vi "AlliGator GUI Actions.vi"(0 "AlliGator Q Elements in":T4[](array[typedef]), 1 "VI in":refnum<vi>, 2 "Script":bool, 5 "AlliGator IV DVR":refnum<data-value>, 7 "AlliGator Q Event in":T5=enum."GUI:Idle", 9 "Data":variant, 11 "error in (no error)":errorcluster, 12 "AlliGator Ctrl Refnums":T6) -> (3 "Script?":bool, 4 "AlliGator Q Elements out":T4[](array[typedef]), 6 "AlliGator IV DVR":refnum<data-value>, 10 "[Notebook Message]":T1[](array[typedef]) {"Message Style"."Text Alignment" items=["Left", "Right", "Center"]}, 14 "Quit?":bool, 15 "error out":errorcluster)   [LabVIEW 2021, in "AlliGator Action Engine.lvlib"]
doc: "Processes AlliGator GUI-related actions."
uses:
  AlliGator Action Engine.lvlib
  AlliGator Displayed Image.ctl
  AlliGator Source Image.lvlib
  Alligator Elements Order in Action Stack.ctl
  AlliGator Q Event.ctl
  AlliGator Q Element.ctl
  AlliGator GUI.lvlib
  AlliGator Variables List.ctl
  AlliGator Globals, Variables & Constants.lvlib
  Variant/Variant to Data/Variant to Data.lvlib
  Variant/Variant to Data/Variant to U16.vi
  AlliGator Internal Variables.lvlib
  GUI/Embedded Progress Bar Q Element.ctl
  GUI/GUI.lvlib
  AlliGator ROIs.lvlib
  Rich Text Box/Rich Text Box.lvlib
  Strings/Strings.lvlib
  AlliGator Settings.lvlib
  Notebook/Notebook.lvlib
  AlliGator Scripts.lvlib
  Variant/Variant to Data/Variant to Boolean.vi
  AlliGator Settings List.ctl
  AlliGator Abort.vi
  AlliGator State Indicators List.ctl
  AlliGator Set State Indicator Data.ctl
  AlliGator Globals.vi
  Variant/Variant to Data/Variant to String.vi
  AlliGator Python Plugins.lvlib
  Fits/Abort Fit Global.vi
  Fits/Fits.lvlib
  Utilities/Utilities.lvlib
  GUI/Open VI Options.ctl
  AlliGator Windows List.ctl
  AlliGator Open Wndow Event Data.ctl
  Sound/Sound.lvlib
  Formula/Formula.lvlib
  Variant/Variant to Data/Variant to I32.vi
  Test Suites/AlliGator Test Data.ctl
  Test Suites/AlliGator Test Suite.lvlib
  Phasor/Phasor Reference Series.ctl
  Phasor/Phasor.lvlib
  Phasor/Calibration Phasor (m, phi).ctl
  Phasor/Phasor (g, s).ctl
  <vilib>/vision/Image Controls.llb/IMAQ Image.ctl
  Image/Named ROI Description.ctl
  Image/Image.lvlib
  AlliGator Baseline Subtraction Method.ctl
  AlliGator Decay Preprocessing.lvlib
  AlliGator Decay Background Subtraction Info.ctl
  Graphs/XY Graph/XY Graph Plot Shift Method.ctl
  Graphs/XY Graph/XY Graph Add-Ons.lvlib
  Graphs/XY Graph/XY Graph Plot Shift Parameters.ctl
  AlliGator Decay Extrapolation Parameters.ctl
  AlliGator Decay Metadata v3.ctl
  AlliGator Phasor Graph.lvlib
  AlliGator Raw Phasor Plot Data v4.ctl
  AlliGator Data Series Type.ctl
  AlliGator Files.lvlib
  AlliGator Gate Image Set.ctl
  AlliGator FLI Dataset Type.ctl
  Phasor/Phasor Harmonic Data.ctl
  AlliGator Phasor Multi-Harmonic Data.ctl
  AlliGator Phasor Plot.lvlib
  Fits/IRF(X)PSED/Decay Fit Parameters & Derived Quantities List.ctl
  Fits/IRF(X)PSED/Decay Fit Parameters In List.ctl
  AlliGator Decay Fit Parameter Constraints 2.ctl
  AlliGator Decay Fit.lvlib
  Fits/Decay Convolution/Decay Model.ctl
  Fits/Residual Type.ctl
  Fits/IRF(X)PSED/Fit Weights Type.ctl
  Fits/Fit Calculation Method.ctl
  Fits/Non-linear Fitting Algorithm.ctl
  AlliGator Decay Fit Options & Parameters v2.ctl
  AlliGator Decay Fit Parameter Map.lvlib
  AlliGator Gate Arithmetic.ctl
  AlliGator Internal Variables v2.ctl
  AlliGator Registered Events Ctrl Refnums.ctl
  AlliGator Dataset Ctrl Refnums.ctl
  Phasor/Phasor Calibration Type.ctl
  AlliGator Phasor Graph Ctrl Refnums.ctl
  AlliGator Phasor Plot Ctrl Refnums.ctl
  AlliGator State Indicator.ctl
  AlliGator Other Ctrl Refnums.ctl
  AlliGator Image Histogram Control Refnums.ctl
  AlliGator Decay Fit Map Control Refnums.ctl
  AlliGator Ctrl Refnums.ctl
  Rich Text Box/Text Colors.ctl
  Rich Text Box/Text Formatting.ctl
  AlliGator Dataset Channel.ctl
  AlliGator Dual-Channel Datasets.lvlib
  Histograms/Histogram Bin Position.ctl
  Histograms/Histogram Window.lvlib
  Histograms/Histogram Bin Option.ctl
  Histograms/Linear Histogram Options.ctl
  AlliGator Decay Preprocessing Parameters.ctl
  Phasor/Phasor Standard Deviation Options.ctl
  Phasor/Phasor Calibration Map v2.ctl
  Fits/Non-linear Fitting Method v2.ctl
  Fits/IRF(X)PSED/Decay Fit Options v2.ctl
  Fits/IRF(X)PSED/MLE Baseline Offset Type.ctl
  Notebook/Notebook Message Object.ctl
  AlliGator Parameter Maps Data.ctl
  AlliGator Main Window Tabs.ctl
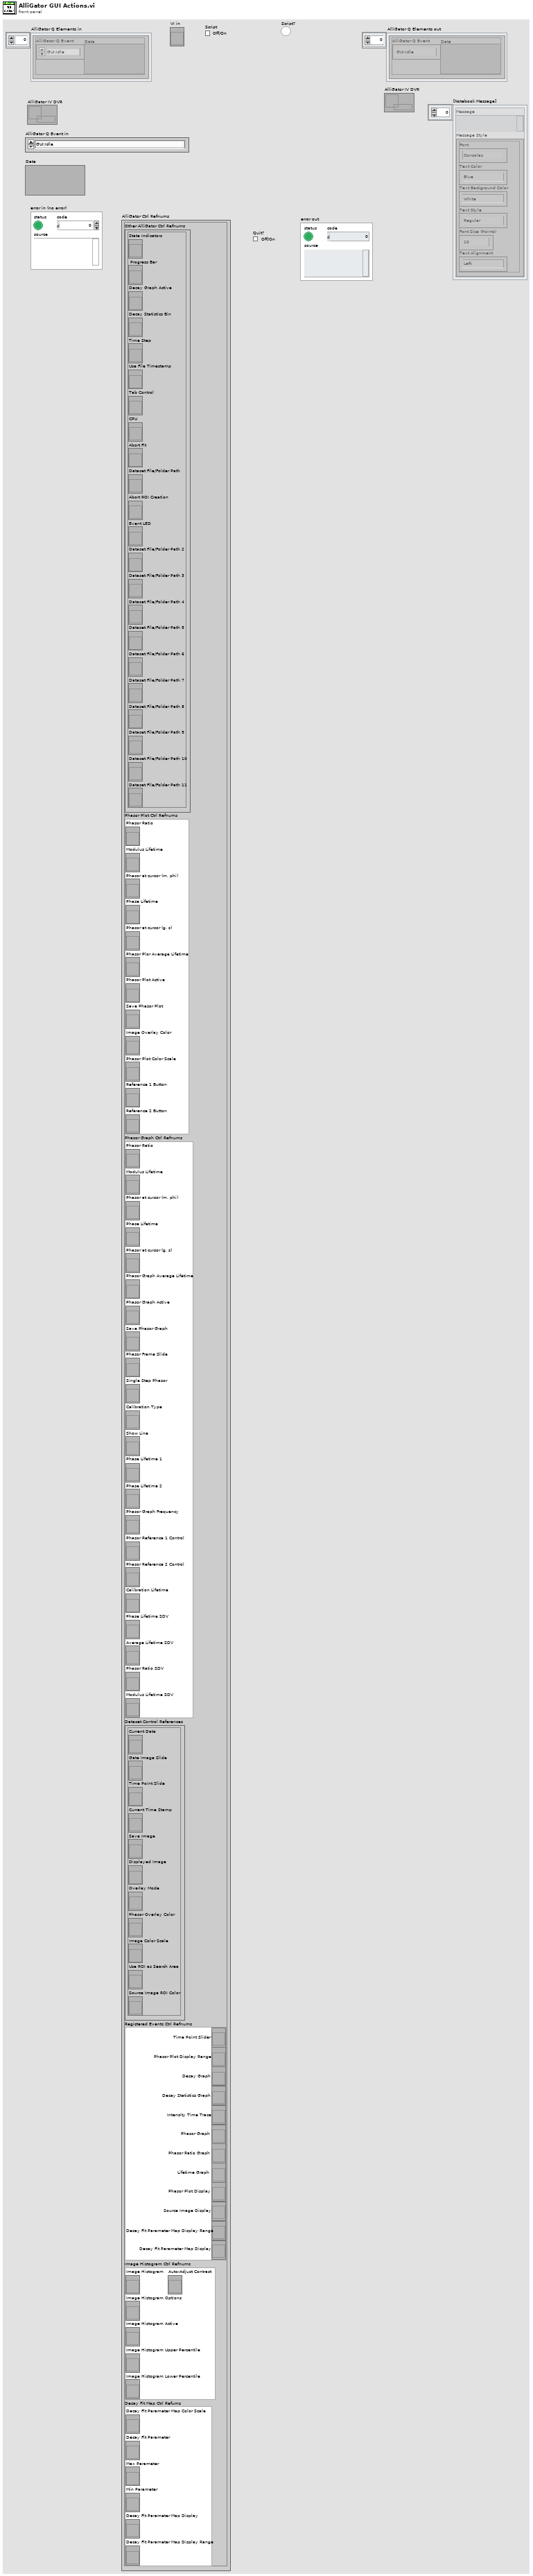
[diagram p1: front panel]
types:
  T1 = typedef "Notebook.lvlib/Notebook Message Object.ctl" = cluster{"Message":string, "Message Style":T2}
  T2 = typedef "Rich Text Box.lvlib/Text Formatting.ctl" = cluster{"Font":string, "Text Color":T3, "Text Background Color":T3, "Text Style":enum16{"Regular", "Bold", "Italic", "Underline", "Strikeout"}, "Font Size (Points)":dbl, "Text Alignment":i32}
  T3 = typedef "Rich Text Box.lvlib/Text Colors.ctl" = enum16{"Unchanged", "Black", "Blue", "Brown", "Gray", "Green", "Orange", "Pink", "Red", "White"}
  T4 = typedef "AlliGator Action Engine.lvlib/AlliGator Q Element.ctl" = cluster{"AlliGator Q Event":T5, "Data":variant}
  T5 = typedef "AlliGator Action Engine.lvlib/AlliGator Q Event.ctl" = enum16{"---- Files ----", "Files:Set Batch Export Files To Save", "Files:Set Dataset Loading & Pre-processing Options", "Files:Check #Frames in Dataset", "Files:Increment Frame Index", "Files:Open Mask Image", "Files:Open White Light Image", "Files:Open Single Dataset", "Files:New Folder of Folders Selected", "Files:Load File (all Types)_Scriptable", "Files:Move Flattened Series to Folders Series", "Files:Select Folder", "Files:Load FLI Dataset", "Files:Load Swiss SPAD 1 Dataset", "Files:Load Swiss SPAD 2 Dataset", "Files:Load .sdt FLI Dataset", "Files:Load .ptu FLI Dataset", "Files:Load .bin FLI Dataset", "Files:Load Single Gate Image Folder", "Files:Load I/m/phi Dataset (deprecated)", "Files:Load Single Image", "Files:Subtract Background File", "Files:Export FLI Dataset", "Files:Load HDF5 FLI Dataset", "Files:Set Destination File Path", "Files:Save Mask Image", "Files:Batch Conversion", "Files:New Folder Selected", "Files:Close FLI Dataset", "Files:Close FLI Dataset Series", "Files:Close White Light Image", "Files:Close Mask Image", "---- FLI Dataset ----", "FLI Dataset:Channel Arithmetic", "FLI Dataset:Export Average Lifetime Map as ASCII", "FLI Dataset:Export User-Defined Quantity Map as ASCII", "FLI Dataset:Python Function FLI Dataset Event", "FLI Dataset:ROI Analysis", "FLI Dataset:Tilted Logistic Square Gated IRF Characteristics Map", "FLI Dataset:Logistic Square Gated IRF Characteristics Map", "FLI Dataset:Square Gated IRF Characteristics Map", "FLI Dataset:Multi-ROI Single-Pixel Phasor Analysis", "FLI Dataset:Multi-ROI Single-Pixel NLSF Analysis", "FLI Dataset:All ROIs IRF Extraction", "FLI Dataset:All ROIs Decay Fit Non-Interactive (Fast + Individual IRF)", "FLI Dataset:All ROIs Phasor Analysis", "FLI Dataset:All ROIs Decay Fit", "FLI Dataset:Fluorescence Decay Statistics", "FLI Dataset:Update Decay Statistics Graph", "FLI Dataset:Get Decay from ROI", "FLI Dataset:All ROIs Average Lifetimes", "---- FLI Dataset Series ----", "FLI Dataset Series:Sum All Datasets in Series", "FLI Dataset Series:Add Dataset to Accumulated Dataset", "FLI Dataset Series:Display Accumulated Dataset", "FLI Dataset Series:Clear Dataset Series Sum", "FLI Dataset Series:Time-Series Analysis (NLSF)", "FLI Dataset Series:Time-Series Analysis (Phasor)", "---- Image ----", "Image:Update Image Profile Plots", "Image:Image Histogram Cursor Move", "Image:Image Histogram", "Image:Image Contrast", "Image:Set Image Histogram Cursor Move Flag", "Image:Clear Image Overlay", "Image:Use ROI as Search Area", "Image:Set ROI Diameter", "Image:Save Image Data as TIFF", "Image:Save Displayed Image with Overlay", "Image:Save Image Overlay Only", "Image:Save Image as Hot Pixel Mask", "Image:Change Source Image Color Palette", "Image:Copy Image to Clipboard", "Image:Source Image ROI Selection", "Image:Delete All ROIs", "Image:Delete All Unselected ROIs", "Image:Delete ROI", "Image:Merge All ROIs", "Image:Store ROI", "Image:Source Image ROI Storage", "Image:Export ROI Description to Notebook", "Image:Save ROI", "Image:Load ROI", "Image:Paste ROI Definition", "Image:Clear ROI", "Image:Identify ROIs in Mask Image", "Image:Create Complementary ROI", "Image:Create Contour ROI", "Image:Create ROI(s) from Pixels with Peak above Min_Scriptable", "Image:Create ROI(s) from Pixels with Intensity above Min_Scriptable", "Image:Compute ROI Statistics", "Image:Delete ROI(s) based on ROI Characteristics", "Image:Create ROI Grid", "Image:ROI to Individual Pixel ROIs", "Image:Python Function Source Image Event", "Image:Show Phasor Calibration Map ROI Centers", "Image:Convert ROI to Mask Image", "Image:Mouse Move", "Image:Mouse Up", "Image:Set Source Image Mouse Move Flag", "Image:Add Scale Bar Overlay", "Image:Delete Existing ROIs Option", "---- Decay ----", "Decay:Clear IRF/Reference Plot", "Decay:Clear Local IRFs", "Decay:Add Decay to Graph", "Decay:Smoothen Plot", "Decay:Smoothen Plot Tail", "Decay:Average Selected Plots", "Decay:Extract IRF", "Decay:Optimal IRF Extraction", "Decay:Threshold IRF", "Decay:Fit to Model IRF", "Decay:Fit IRF to Square Gate", "Decay:Fit IRF to Logistic Square Gate", "Decay:Fit IRF to Tilted Logistic Square Gate", "Decay:Create Bounding Cursors Set", "Decay:Export Bounding Cursors Definition to Notebook", "Decay:Denoise Plot", "Decay:Compute Cumulative Function", "Decay:Use as Reference Decay", "Decay:Show Reference Decay/IRF", "Decay:Extrapolate Decay", "Decay:Create Head & Tail Bounding Cursors", "Decay:Store Cursor-defined Head & Tail Fractions", "Decay:Rebin Plot", "Decay:1-Normalize Decay", "Decay:[0-1]-Normalize Plot", "Decay:Straighten Decay", "Decay:Shift Decay", "Decay:Fold Decay", "Decay:Fit Decay", "Decay:Global Fit of Selected Decays", "Decay:Post Global Fit Script", "Decay:Add Global Fit Parameters to Graph", "Decay:Add Decay Parameter(s) to Plot (Graph)", "Decay:Export Decay to Phasor Graph", "Decay:Plot Decay Shifts", "Decay:Compute Average Lifetime", "Decay:Plot Convolution", "Decay:Graph Tip Strip Update", "---- Decay Statistics ----", "Decay Statistics:Tip Strip Update", "---- Intensity Time Trace ----", "Intensity Time Trace:Use File Timestamp", "Intensity Time Trace:Load Intensity Corrections File", "Intensity Time Trace:Clear Intensity Corrections File", "Intensity Time Trace:Tip Strip Update", "---- Phasor Plot ----", "Phasor Plot:Build Phasor Plot", "Phasor Plot:Change Phasor Plot Color Palette", "Phasor Plot:Adjust Phasor Plot Display Range", "Phasor Plot:Highlight Image ROI in Phasor Plot", "Phasor Plot:Save Phasor Plot Image with Overlay", "Phasor Plot:Export Complex Phasor Map", "Phasor Plot:Export Phasor Ratio Map", "Phasor Plot:Export Average Lifetime Map", "Phasor Plot:Compute Phase Lifetime Histogram", "Phasor Plot:Compute Phasor Ratio Histogram", "Phasor Plot:Compute Phase Lifetime vs Intensity Scatter Plot", "Phasor Plot:Weber 2-Component Decomposition", "Phasor Plot:Update Phasor Color Map Vertices", "Phasor Plot:Clear Phasor Overlay", "Phasor Plot:Use Segment Extremities as References", "Phasor Plot:Use UC/Segment Intersections as References", "Phasor Plot:Use UC/Principal Axis Intersections as References", "Phasor Plot:Use UC/Linear Fit Intersections as References", "Phasor Plot:Update Phasor Plot Reference", "Phasor Plot:Show Local Phasor Info in Phasor Plot", "Phasor Plot:Update Phasor Plot State", "Phasor Plot:Phasor Plot ROI Storage", "Phasor Plot:Phasor Plot ROI Selection", "Phasor Plot:Python Function Phasor Plot Event", "Phasor Plot:Overlay Phasor ROI, Ratio or Map in Source Image", "Phasor Plot:Compute Decay of Selected Phasors", "Phasor Plot:Phasor at Image Pixel", "Phasor Plot:Mouse Move", "Phasor Plot:Mouse Up", "Phasor Plot:Display Range Mouse Move", "Phasor Plot:Set Mouse Move Flag", "---- Phasor Graph ----", "Phasor Graph:Calibrated Phasor Map Series", "Phasor Graph:Whole Image Phasor Scatter Plot (Todo)", "Phasor Graph:Get Phasor Value", "Phasor Graph:Create New Phasor Plot Dialog", "Phasor Graph:Update Last Phasor Value", "Phasor Graph:Update Phasor (m, phi)", "Phasor Graph:Remove Single Phasor from Plot", "Phasor Graph:Add Single Phasor to Plot", "Phasor Graph:Remove Phasor Plot", "Phasor Graph:Remove Selected Phasor Plots", "Phasor Graph:Clear Phasor Data", "Phasor Graph:Clear Phasor Graph", "Phasor Graph:Cursor Move", "Phasor Graph:Draw Cursor Connecting Line", "Phasor Graph:Clear Cursor Connecting Line", "Phasor Graph:Find UC Intersection", "Phasor Graph:Use UC/Cursor-Defined Line Intersections", "Phasor Graph:Use Selected Plots Fitted Line/UC Intersections", "Phasor Graph:Use Selected Plots Principal Axis/UC Intersections", "Phasor Graph:Show Single Phasor", "Phasor Graph:Save Single Phasor Plot", "Phasor Graph:Save All Phasor Plots", "Phasor Graph:Load Phasor Plot(s)", "Phasor Graph:Phasor Multiplication", "Phasor Graph:Compute Average Phasor", "Phasor Graph:Compute Multiple Average Phasors (Selected Plots)", "Phasor Graph:Export Single Phasor Plot Phase Lifetimes", "Phasor Graph:Phase Lifetime Trajectory", "Phasor Graph:Phase Lifetime vs Intensity Scatter Plot (deprecated)", "Phasor Graph:Parameter 2 vs Parameter 1 Scatter Plot", "Phasor Graph:Use Cursor n Location", "Phasor Graph:Set Reference n to Current Phase Lifetime Value", "Phasor Graph:Set Reference n to Lifetime Value", "Phasor Graph:Set Cursor n Location", "Phasor Graph:Save Phasor Graph Image", "Phasor Graph:Update SEPL Plot", "Phasor Graph:Export Single Phasor Plot Data", "Phasor Graph:Export Selected Phasor Plots Data", "Phasor Graph:Python Function Phasor Graph Event", "Phasor Graph:Tip Strip Update", "---- Calibration ----", "Calibration:Set Calibration Type", "Calibration:Load/Save Phasor Calibration", "Calibration:Load/Save Phasor Calibration Series", "Calibration:Load/Save Phasor Calibration Map", "Calibration:Use as Calibration", "Calibration:Compute Optimal Calibration from Phasor References", "Calibration:Clear Phasor Calibration", "Calibration:Single Phasor Calibration Information", "Calibration:Use as Calibration Series", "Calibration:Use as Calibration Map", "Calibration:Clear Calibration Series", "Calibration:Phasor Calibration Series Information", "Calibration:Clear Calibration Map", "Calibration:Phasor Calibration Map Information", "Calibration:Apply Phasor Calibration", "Calibration:Update Single Plot Calibration", "Calibration:Update Multiple Plots Calibration", "Calibration:Clear Single Plot Calibration", "Calibration:Clear All Plots Calibrations", "Calibration:Clear Plot(s) Calibration(s)?", "Calibration:Phasor Calibration Maps (# Gates Series)", "---- Phasor Ratio ----", "Phasor Ratio:Clear Reference n", "Phasor Ratio:Toggle Selected Plot(s)  Lock to Reference 1", "Phasor Ratio:Use as Reference n", "Phasor Ratio:Send Reference n to Notebook", "Phasor Ratio:Toggle Selected Plot(s)  Lock to Reference 2", "Phasor Ratio:Compute Phasor Ratio at Mouse Location", "Phasor Ratio:Compute Phasor Plot's Average Phasor Ratio", "Phasor Ratio:Compute Time-Series Phasor Ratios", "Phasor Ratio:Fit Line to Phasor Ratio Plot", "Phasor Ratio:Save References", "Phasor Ratio:Load References", "Phasor Ratio:Update Phasor Reference 1", "Phasor Ratio:Update Phasor Reference 2", "Phasor Ratio:Move Cursor n to Reference n", "Phasor Ratio:Use as Phasor Reference 1 Lifetime", "Phasor Ratio:Use as Phasor Reference 2 Lifetime", "Phasor Ratio:Export Phasor Ratio Map as ASCII", "Phasor Ratio:Tip Strip Update", "---- Lifetime & Other Parameters Graph ----", "Lifetime:Tip Strip Update", "---- Decay Fit Parameter Map ----", "Decay Fit Parameter Map:Export ROI NLSF Data as ASCII", "Decay Fit Parameter Map:Set Decay Fit  Parameter Map Selection", "Decay Fit Parameter Map:Build Decay Fit Parameter Map", "Decay Fit Parameter Map:Change Decay Fit Parameter Map Color Palette", "Decay Fit Parameter Map:Export Decay Fit Parameter Map Data as ASCII", "Decay Fit Parameter Map:Export All Decay Fit Parameter Maps Data as ASCII", "Decay Fit Parameter Map:Send Map Data to Lifetime Graph", "Decay Fit Parameter Map:Save Decay Fit Parameter Map Image", "Decay Fit Parameter Map:Save-Load IRFs & Fit Data", "Decay Fit Parameter Map:Update Local Decay Plots", "Decay Fit Parameter Map:Python Function Decay Fit Parameters Map Event", "Decay Fit Parameter Map:Overlay Decay Fit Parameter Map in Source Image", "Decay Fit Parameter Map:Plot Map Data vs Intensity", "Decay Fit Parameter Map:Mouse Up", "Decay Fit Parameter Map:Display Range Mouse Move", "---- Generic Graph ----", "Generic Graph:Generic XY Graph Event", "Generic Graph:Python Function XY Graph Event", "Generic Graph:New Plot", "Generic Graph:Save Plot", "Generic Graph:XY Plot Histogram", "Generic Graph:Set XY Graph Plot Name", "Generic Graph:Set Last Cursor Style", "Generic Graph:Tip Strip Update", "---- GUI ----", "GUI:Start Script", "GUI:Type of Displayed Image Changed", "GUI:Gate Image Slide Changed", "GUI:Show Busy Icon", "GUI:Show Busy Icon & Abort Button", "GUI:Hide Busy Icon", "GUI:Hide Busy Icon & Abort Button", "GUI:Abort", "GUI:End Script", "GUI:Start Timing", "GUI:End Timing", "GUI:Set State Indicator", "GUI:Send Parameters JSON Strings to Clipboard", "GUI:Set Gate Step", "GUI:Idle", "GUI:Initialization", "GUI:Quit", "GUI:Increment Dataset Index", "GUI:Set Dataset Index to -1", "GUI:Time Series Slider Moved", "GUI:Time Series Slider Changed", "GUI:Toggle Playback or Loop", "GUI:Playback Script", "GUI:Set Phasor Frequency", "GUI:Open Window", "GUI:Start Test Script", "GUI:End Test Script", "DEBUG"}
  T6 = typedef "AlliGator GUI.lvlib/AlliGator Ctrl Refnums.ctl" = cluster{"Other AlliGator Ctrl Refnums":T7, "Phasor Plot Ctrl Refnums":T8, "Phasor Graph Ctrl Refnums":T9, "Dataset Control References":T10, "Registered Events Ctrl Refnums":T11, "Image Histogram Ctrl Refnums":T12, "Decay Fit Map Ctrl Refums":T13}
  T7 = typedef "AlliGator GUI.lvlib/AlliGator Other Ctrl Refnums.ctl" = cluster{"State Indicators":refnum<vi>, " Progress Bar":refnum<vi>, "Decay Graph Active":refnum<vi>, "Decay Statistics Bin":refnum<vi>, "Time Step":refnum<vi>, "Use File Timestamp":refnum<vi>, "Tab Control":refnum<vi>, "CPU":refnum<vi>, "Abort Fit":refnum<vi>, "Dataset File/Folder Path":refnum<vi>, "Abort ROI Creation":refnum<vi>, "Event LED":refnum<vi>, "Dataset File/Folder Path 2":refnum<vi>, "Dataset File/Folder Path 3":refnum<vi>, "Dataset File/Folder Path 4":refnum<vi>, "Dataset File/Folder Path 5":refnum<vi>, "Dataset File/Folder Path 6":refnum<vi>, "Dataset File/Folder Path 7":refnum<vi>, "Dataset File/Folder Path 8":refnum<vi>, "Dataset File/Folder Path 9":refnum<vi>, "Dataset File/Folder Path 10":refnum<vi>, "Dataset File/Folder Path 11":refnum<vi>}
  T8 = typedef "AlliGator GUI.lvlib/AlliGator Phasor Plot Ctrl Refnums.ctl" = cluster{"Phasor Ratio":refnum<vi>, "Modulus Lifetime":refnum<vi>, "Phasor at cursor (m, phi)":refnum<vi>, "Phase Lifetime":refnum<vi>, "Phasor at cursor (g, s)":refnum<vi>, "Phasor Plor Average Lifetime":refnum<vi>, "Phasor Plot Active":refnum<vi>, "Save Phasor Plot":refnum<vi>, "Image Overlay Color":refnum<vi>, "Phasor Plot Color Scale":refnum<vi>, "Reference 1 Button":refnum<vi>, "Reference 2 Button":refnum<vi>}
  T9 = typedef "AlliGator GUI.lvlib/AlliGator Phasor Graph Ctrl Refnums.ctl" = cluster{"Phasor Ratio":refnum<vi>, "Modulus Lifetime":refnum<vi>, "Phasor at cursor (m, phi)":refnum<vi>, "Phase Lifetime":refnum<vi>, "Phasor at cursor (g, s)":refnum<vi>, "Phasor Graph Average Lifetime":refnum<vi>, "Phasor Graph Active":refnum<vi>, "Save Phasor Graph":refnum<vi>, "Phasor Frame Slide":refnum<vi>, "Single Step Phasor":refnum<vi>, "Calibration Type":refnum<vi>, "Show Line":refnum<vi>, "Phase Lifetime 1":refnum<vi>, "Phase Lifetime 2":refnum<vi>, "Phasor Graph Frequency":refnum<vi>, "Phasor Reference 1 Control":refnum<vi>, "Phasor Reference 2 Control":refnum<vi>, "Calibration Lifetime":refnum<vi>, "Phase Lifetime SDV":refnum<vi>, "Average Lifetime SDV":refnum<vi>, "Phasor Ratio SDV":refnum<vi>, "Modulus Lifetime SDV":refnum<vi>}
  T10 = typedef "AlliGator GUI.lvlib/AlliGator Dataset Ctrl Refnums.ctl" = cluster{"Current Data":refnum<vi>, "Gate Image Slide":refnum<vi>, "Time Point Slide":refnum<vi>, "Current Time Stamp":refnum<vi>, "Save Image":refnum<vi>, "Displayed Image":refnum<vi>, "Overlay Mode":refnum<vi>, "Phasor Overlay Color":refnum<vi>, "Image Color Scale":refnum<vi>, "Use ROI as Search Area":refnum<vi>, "Source Image ROI Color":refnum<vi>}
  T11 = typedef "AlliGator GUI.lvlib/AlliGator Registered Events Ctrl Refnums.ctl" = cluster{"Time Point Slider":refnum<vi>, "Phasor Plot Display Range":refnum<vi>, "Decay Graph":refnum<vi>, "Decay Statistics Graph":refnum<vi>, "Intensity Time Trace":refnum<vi>, "Phasor Graph":refnum<vi>, "Phasor Ratio Graph":refnum<vi>, "Lifetime Graph":refnum<vi>, "Phasor Plot Display":refnum<vi>, "Source Image Display":refnum<vi>, "Decay Fit Parameter Map Display Range":refnum<vi>, "Decay Fit Parameter Map Display":refnum<vi>}
  T12 = typedef "AlliGator GUI.lvlib/AlliGator Image Histogram Control Refnums.ctl" = cluster{"Image Histogram":refnum<vi>, "Image Histogram Options":refnum<vi>, "Image Histogram Active":refnum<vi>, "Image Histogram Upper Percentile":refnum<vi>, "Image Histogram Lower Percentile":refnum<vi>, "Auto-Adjust Contrast":refnum<vi>}
  T13 = typedef "AlliGator Decay Fit Parameter Map.lvlib/AlliGator Decay Fit Map Control Refnums.ctl" = cluster{"Decay Fit Parameter Map Color Scale":refnum<vi>, "Decay Fit Parameter":refnum<vi>, "Max Parameter":refnum<vi>, "Min Parameter":refnum<vi>, "Decay Fit Parameter Map Display":refnum<vi>, "Decay Fit Parameter Map Display Range":refnum<vi>}
  T14 = typedef "AlliGator Globals, Variables & Constants.lvlib/AlliGator Variables List.ctl" = enum16{"---- GUI ----", "GUI:Initialization Status", "GUI:State Indicators Refnum", "GUI:Original AlliGator Menu Items", "GUI:Current Action Loop State", "GUI:Script in progress", "GUI:Playback", "GUI:Loop Playback", "GUI:Search ROI Used", "GUI:Search ROI", "Decay Graph Max Legend Size", "Intensity Graph Max Legend Size", "Decay Statistics Graph Max Legend Size", "Phasor Graph Max Legend Size", "Phasor Ratio Graph Max Legend Size", "Lifetime Graph Max Legend Size", "---- Files ----", "Files:Export Dataset Frames as Individual Files", "Files:Show Batch Export Help Balloons", "Files:Frames in Dataset", "Files:ptu File Frame Start Indices", "Files:Current Frame in Dataset", "Files:Current Frame Timestamp", "Files:Dataset Loaded", "Files:Dataset Metadata", "Files:Dataset Channel", "Files:Dataset Data Description", "Files:Background Dataset Metadata", "Files:Background Dataset Channel", "Files:Background Dataset Data Description", "Files:Background File Subtraction", "Files:Background File Path", "Files:Background File Pile-up Correction", "Files:Background File Pixel Well Capacity", "Files:Background File Scaling Factor", "Files:Current Dataset Load Settings", "Files:Dataset Path", "Files:ICCD-specific Information", "Files:Macrotime Gate Separation", "------ Python Plugins ------", "Python Plugins:Information", "Python Plugins:Python Session", "Python Plugins:Valid Python Session?", "---- Source Image ----", "Source Image:ROIs", "Source Image:Current ROI", "Source Image:ROI Event Refnum", "X_Source Image Display Range", "X_Source Image Palette Information", "X_Type of Displayed Image", "X_Time Gate Slider", "Source Image:Palette List", "Source Image:Scale", "Source Image:ROI Overlay Color", "Source Image:Overlay to Erase", "Source Image:Is Displayed Image Accumulated", "Source Image:White Light Image Modified", "Source Image:Mask Image Modified", "---- Image Profile Window ----", "Image Profile:Overlay ROI in Source Image", "Image Profile:Window Event Refnum", "Image Profile:IntensityType", "Image Profile:Intensity Average Type", "Image Profile:Intensity-weighted SDV", "Image Profile:Box Profile Type", "Image Profile:Window Open", "Image Profile:Plotted Fit Parameter", "------ Phasor Graph -------", "Phasor Graph:Show Line", "---- Phasor Plot ---", "Phasor Plot:Parameters Changed", "Phasor Plot:FLI Dataset Modified since last Calculation", "Phasor Harmonics Data", "Selected Phasor Harmonics", "Phasor Harmonic Manager Event Refnum", "Phasor Plot:ROIs", "Phasor Plot:Current ROI", "Phasor Plot:ROI Event Refnum", "Phasor Plot:Image Reference Points", "Phasor Plot:Computed", "Phasor Plot:Palette Information", "Phasor Plot:Palette List", "Phasor Plot:Phasor Ratio Palette Information", "Phasor Plot:Phasor Ratio Palette List", "Phasor Plot:Image Scale", "Phasor Plot:Image Overlay to Erase", "Phasor Plot:Image Elements to Update", "Phasor Plot:Current Calculation Parameters", "Phasor Plot:Current Calibration Options", "Phasor Plot:Reset Cumulated Phasor Plot", "Phasor Plot:Reference 1", "Phasor Plot:Lifetime Reference 1", "Phasor Plot:Reference 1 Frequency", "Phasor Plot:Reference 2", "Phasor Plot:Lifetime Reference 2", "Phasor Plot:Reference 2 Frequency", "---- Decay Analysis ----", "Number of Selected Decays to Fit", "LS Fit Results", "LAR Fit Results", "BS Fit Results", "Last Decay Max - Min", "Best Fit Parameters", "Best Fit Parameter Names", "Actual Size X", "Actual Size Y", "Binning X", "Binning Y", "Actual # Gates", "Dataset Number", "Gates to...", "Gates Skipped", "Gates to keep", "Gate Step", "Gate Separation", "Reversed Gates", "Pile-up Correction", "Pixel Well Capacity", "Background Subtracted", "Background Subtraction Method", "Background Definition Range", "Background File (deprecated)", "Number of Dataset Accumulated", "Array of Accumulated Dataset Paths", "Do Averaged Datasets", "Destination File Path", "Process Plot Target", "Use 1/D as Phasor Frequency", "---- Decay Fit Parameter Map -----", "Decay Fit Parameter Map:Palette Information", "Decay Fit Parameter Map:Palette List", "------- Local Decay Window ---------", "Local Decay Graph Window:Event Refnum", "Local Decay Graph Window:Use normalized IRF for convolution", "----- Miscellaneous ----", "Misc:Skippable Dialog Windows Status"}
  T15 = typedef "AlliGator Settings.lvlib/AlliGator Settings List.ctl" = enum16{"GUI:Visible Settings Tab", "GUI:Last Run Version", "Source Image:Use Image Histogram for Contrast", "Source Image:Low Count Pixels Rejection Options", "Source Image:High Count Pixels Rejection Options", "Source Image:Use Image Brightness", "Source Image:Blend Overlay with Image Background", "Source Image:Use Fixed ROI Diameter", "Source Image:ROI Diameter", "Source Image:ROI Center Color", "Source Image:Peak Threshold", "Source Image:Intensity Threshold", "Source Image:Image Binning Options", "Source Image:Image Smoothing Options", "Source Image:Image Histogram Active", "Source Image:Invert Binary Mask", "Source Image:Hot Pixel Removal", "Source Image:Overlay Analyzed ROI Center", "Source Image:Auto-Adjust Contrast", "Source Image:Histogram Lower Percentile", "Source Image:Histogram Upper Percentile", "Source Image:Save Source Image", "Source Image:Scale Bar Options", "Source Image:Image Resolution (Pixel Size)", "Source Image:Flatfield Correction", "Source Image:Show Dead Left Columns Correction", "Source Image:Dead Left Columns Correction", "Source Image:Image Pre-Processing Operations Order", "Data Information:Gate Width", "Data Information:Nanotime Gate Separation", "Data Information:Macrotime Gate Separation", "Data Information:Gate Step", "Data Information:# Gates", "Data Information:Gate Image Exposure", "Data Information:Gate Image Integration", "Data Information:Gates to Skip", "Data Information:Gates to Keep", "Data Information:Define Gates to", "Data Information:Channel Name", "Data Information:Available Channel Names", "Data Information:Channel Arithmetic", "Data Information:Background File Subtraction", "Data Information:Background File", "Data Information:Background Scaling Factor", "Data Information:Background Pile-up Correction", "Data Information:Background Pixel Well Capacity", "Data Information:Laser Period", "Data Information:SYNC Period", "Data Information:Pile-up Correction", "Data Information:Pixel Well Capacity", "Data Information:Dataset Scaling Factor", "Fluorescence Decay_Decay Pre-Processing:Reverse Gates", "Fluorescence Decay_Decay Pre-Processing:Verbose Decay Pre-Processing", "Fluorescence Decay_Decay Pre-Processing:Use Decay Pre-Processing", "Fluorescence Decay_Decay Pre-Processing:Background Subtraction", "Fluorescence Decay_Decay Pre-Processing:Background Definition Range", "Fluorescence Decay_Decay Pre-Processing:Baseline Subtraction Method", "Fluorescence Decay_Decay Pre-Processing:Decay Pre-Processing Operations Order", "Fluorescence Decay_Decay Pre-Processing:Smoothing Parameter", "Fluorescence Decay_Decay Pre-Processing:Shift Decay", "Fluorescence Decay_Decay Pre-Processing:Decay Shift Parameters", "Fluorescence Decay_Decay Pre-Processing:Fold Decay", "Fluorescence Decay_Decay Pre-Processing:# Folds", "Fluorescence Decay_Decay Pre-Processing:1-Normalize Decay", "Fluorescence Decay_Decay Pre-Processing:[0-1]-Normalize Decay", "Fluorescence Decay_Decay Pre-Processing:Smoothen Decay", "Fluorescence Decay_Decay Pre-Processing:Extrapolate Decay", "Fluorescence Decay_Decay Pre-Processing:Use Periodicity", "Fluorescence Decay_Decay Pre-Processing:Use Cursors", "Fluorescence Decay_Decay Pre-Processing:Tail Fraction", "Fluorescence Decay_Decay Pre-Processing:Head Fraction", "Fluorescence Decay_Decay Pre-Processing:Additional Points", "Fluorescence Decay_Decay Pre-Processing:Straighten Decay", "Fluorescence Decay_Decay Pre-Processing:Constant Background", "Fluorescence Decay_Decay Pre-Processing:Pixel-Normalize Decay", "Fluorescence Decay_Advanced Analysis:Extract IRF instead of Decay", "Fluorescence Decay_Advanced Analysis:IRF Extraction Options", "Fluorescence Decay_Advanced Analysis:IRF Optimization Options", "Fluorescence Decay_Advanced Analysis:Square Pulse Options", "Fluorescence Decay_Advanced Analysis:IRF Order", "Fluorescence Decay_Advanced Analysis:IRF Time Constants", "Fluorescence Decay_Advanced Analysis:Wavelet Analysis Options", "Fluorescence Decay_Advanced Analysis:Average Lifetime Options", "Fluorescence Decay_Fit Options:Fit Options", "Fluorescence Decay_Fit Options:Use Legacy Fitting Approach", "Fluorescence Decay_Fit Options:Use Data Information Laser Period", "Fluorescence Decay_Fit Parameters:Displayed Fit Parameters", "Fluorescence Decay_Fit Parameters:Fit Parameter Constraints", "Fluorescence Decay_Fit Parameters:Export Tabulated Results", "Fluorescence Decay_Fit Parameters:MLE Baseline Offset Type", "Fluorescence Decay_Fit Parameters:MLE Baseline Offset", "Fluorescence Decay_Fit Parameters:Guess Parameter Names", "Fluorescence Decay_Fit Parameters:Guess Parameter Values", "Fluorescence Decay_Fit Parameters:Guess Parameters Options", "Fluorescence Decay_Styles:Show Last Decay Only", "Fluorescence Decay_Styles:Decay Graph Color Array", "Fluorescence Decay:Decay Graph Active", "Fluorescence Decay Statistics:Min Peak Value", "Fluorescence Decay Statistics:Reject Low Decay Peak Pixels", "Fluorescence Decay Statistics:Reject High Decay Peak Pixels", "Fluorescence Decay Statistics:Max Peak Value", "Time Traces:Use File Timestamp", "Time Traces:Time Step", "Time Traces:Use Intensity Correction File", "Time Traces:Intensity Correction File", "Phasor Plot:Phasor Plot Smoothing Options", "Phasor Plot:Phasor Plot Size", "Phasor Plot:Phasor Plot Graphics Options", "Phasor Plot:Cumulative Phasor Plot", "Phasor Plot:Use Phasor Brightness", "Phasor Plot:Blend Overlay with Phasor Background", "Phasor Plot:Save Phasor Plot", "Phasor Plot:Show References", "Phasor Plot:Phasor Ratio Decay Range", "Phasor Plot:Exponential Fading", "Phasor Plot:Phasor Ratio Reference Colors", "Phasor Plot:Reference Radius", "Phasor Plot:Show Color Map Vertices", "Phasor Plot:Phasor Plot Active", "Phasor Plot:Phasor Ratio Color Map Type", "Phasor Plot:Phasor Ratio Color Map", "Phasor Plot:Phasor Ratio Display Range", "Phasor Plot:Selected Image ROI(s)", "Phasor Plot:All Image ROIs", "Phasor Plot:Selected Phasor Plot ROI(s)", "Phasor Plot:All Phasor Plot ROIs", "Phasor Plot:Phasor Ratio Color-Coded Quantity", "Phasor Plot:Store Phasor Harmonics", "Phasor Plot:Draw Reference Segment", "Phasor Plot:User-Defined Quantity", "Phasor Graph:Phasor Frequency", "Phasor Graph:Phasor Ratio Type", "Phasor Graph:Pixel-level Phasor Computation", "Phasor Graph:Save Phasor Graph", "Phasor Graph:Phasor Graph Active", "Phasor Graph:Phasor SDV Options", "Phasor Calibration:Use Backup Calibration if needed", "Phasor Graph:Define Shortest Lifetime as", "Phasor Calibration:Backup Calibration Type", "Phasor Calibration:Calibration Type", "Phasor Calibration:Calibration Lifetime", "Phasor Calibration:Calibration Map Algorithm", "Single-Exponential Phasor Locus (SEPL):Gate Parameters", "Single-Exponential Phasor Locus (SEPL):User-defined Gate", "Single-Exponential Phasor Locus (SEPL):User-defined IRF", "Single-Exponential Phasor Locus (SEPL):Phasor Parameters", "Single-Exponential Phasor Locus (SEPL):Decay & IRF Parameters", "Single-Exponential Phasor Locus (SEPL):Display Parameters", "Lifetime Analysis:Decay Analysis Parameters", "Lifetime Analysis:Lifetime Map Active", "Plugins:Python Settings", "Miscellaneous:Verbose Mode", "Miscellaneous:Beep after Script", "Miscellaneous:Saved Image File Format", "Miscellaneous:Exported Gate Image Settings", "Miscellaneous:Include Loading in Timing", "Miscellaneous:Verbose Settings Mode", "Miscellaneous:Histogram Options", "Miscellaneous:Beep on Error", "Miscellaneous:# Logical Processors Used", "Miscellaneous:ROI Description Max Characters", "Miscellaneous:Verbose Error Mode", "Miscellaneous:Transparent Mask Color"}
  T16 = typedef "AlliGator Action Engine.lvlib/Alligator Elements Order in Action Stack.ctl" = enum16{"Enqueue 2 AFTER 1", "Enqueue 2 BEFORE 1"}
  T17 = typedef "AlliGator GUI.lvlib/AlliGator Open Wndow Event Data.ctl" = cluster{"AlliGator Windows":T18, "Open Window Options":T19}
  T18 = typedef "AlliGator GUI.lvlib/AlliGator Windows List.ctl" = enum16{"AlliGator Window", "Settings Window", "Notebook Window", "Dataset Information Window", "Source Image ROI Manager Window", "Phasor Plot ROI Manager Window", "Phasor Harmonic Manager Window", "Histogram Window", "Image Profile Window", "Local Decay Window", "About Window", "Batch Conversion Window", "Shot Noise Influence on Average Lifetime", "Fit Method Benchmark", "AlliGator Alias Definition"}
  T19 = typedef "GUI.lvlib/Open VI Options.ctl" = cluster{"Bring To Front (T)":bool, "Start Hidden? (F)":bool, "Activate? (T)":bool}
  T20 = typedef "GUI.lvlib/Embedded Progress Bar Q Element.ctl" = cluster{"Action":string, "Value":dbl}
  T21 = typedef "AlliGator Action Engine.lvlib/AlliGator State Indicators List.ctl" = enum16{"Phasor Calibration Defined", "Phasor Calibration Series Defined", "Phasor Calibration Map Defined", "Phasor Reference 1 Defined", "Phasor Reference 2 Defined", "Lifetime Reference 1 Defined", "Lifetime Reference 2 Defined", "Phasor Calibration Used", "Phasor Calibration Series Used", "Phasor Calibration Map Used", "Dataset Update Needed", "Phasor Plot Update Needed", "Reference/IRF Defined", "Individual IRFs Defined"}
  T22 = typedef "AlliGator GUI.lvlib/AlliGator Set State Indicator Data.ctl" = cluster{"State Indicators List":T21, "ON/OFF":bool, "# Defined IRFs":i32}
  T23 = typedef "AlliGator Source Image.lvlib/AlliGator Displayed Image.ctl" = enum16{"Single Gate", "Sum of All Gates", "Max of All Gates", "Min of All Gates", "-", "White Ligth Image", "Mask Image"}
  T24 = enum16{"Store Test Name", "Store Test Result", "Read Test Result"}
  T25 = typedef "AlliGator Test Suite.lvlib/AlliGator Test Data.ctl" = cluster{"Test String":string, "error":errorcluster, "Status":bool}
  T26 = typedef "AlliGator Files.lvlib/AlliGator Data Series Type.ctl" = enum16{"Not a Supported Series", "Gate Images Folder Series", "SwissSPAD 2 Dataset Series", "B&H FLI Dataset Series", "PicoQuant PTU FLI Dataset Series", "PicoQuant BIN FLI Dataset Series", "Piccolo hist BIN FLI Dataset Series", "HDF5 FLI Dataset Series"}
  T27 = typedef "AlliGator Displayed Image.ctl" = enum16{"Single Gate", "Sum of All Gates", "Max of All Gates", "Min of All Gates", "-", "White Ligth Image", "Mask Image"}
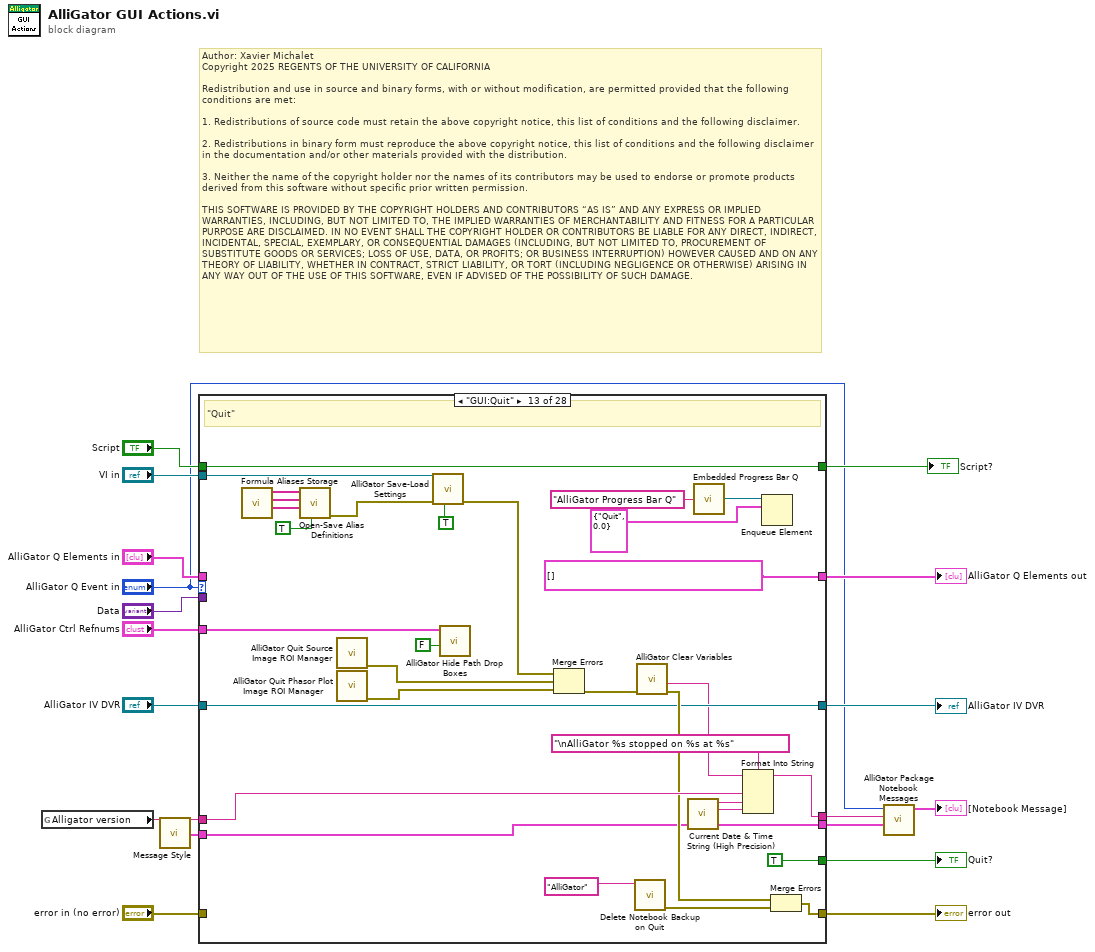
[diagram p0: block diagram]
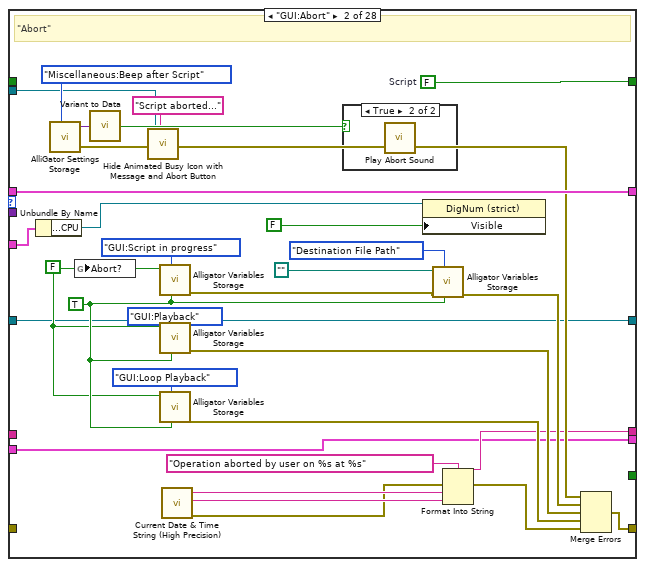
[diagram p3: hidden frame]
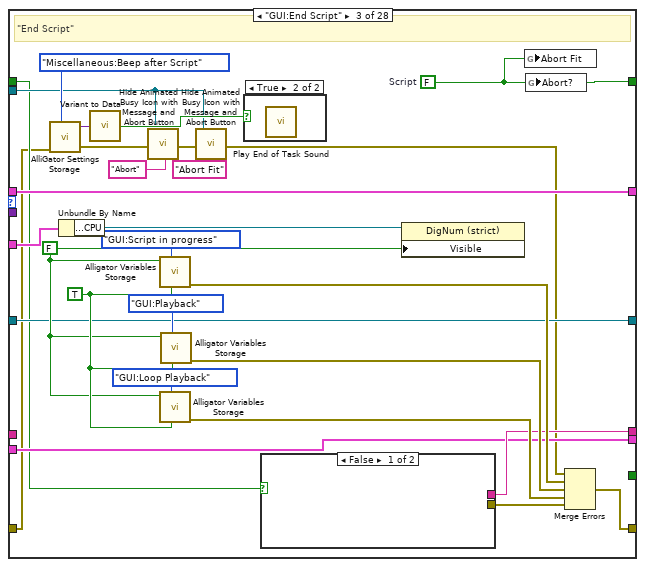
[diagram p5: hidden frame]
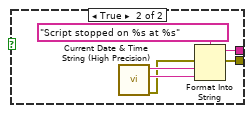
[diagram p6: hidden frame]
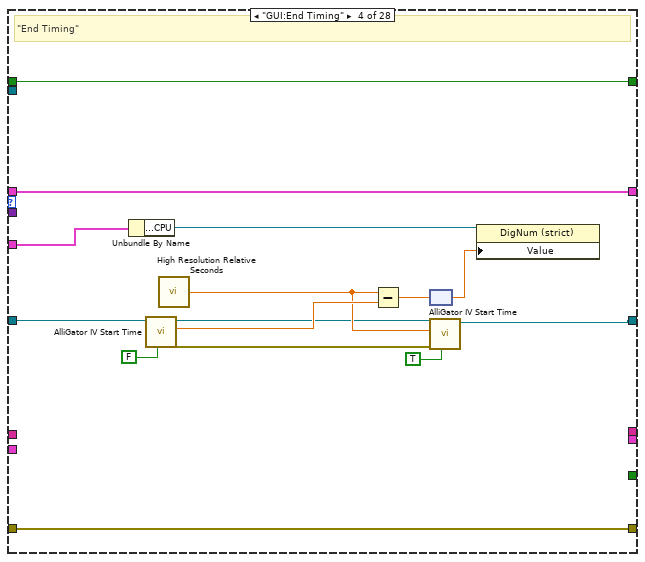
[diagram p8: hidden frame]
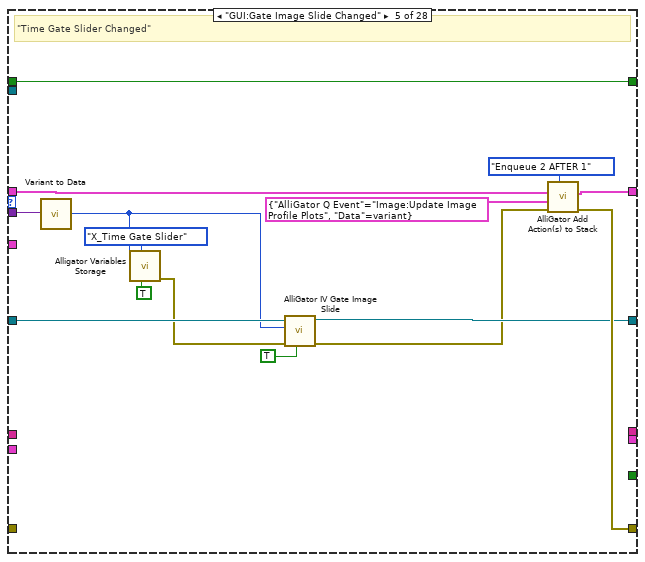
[diagram p9: hidden frame]
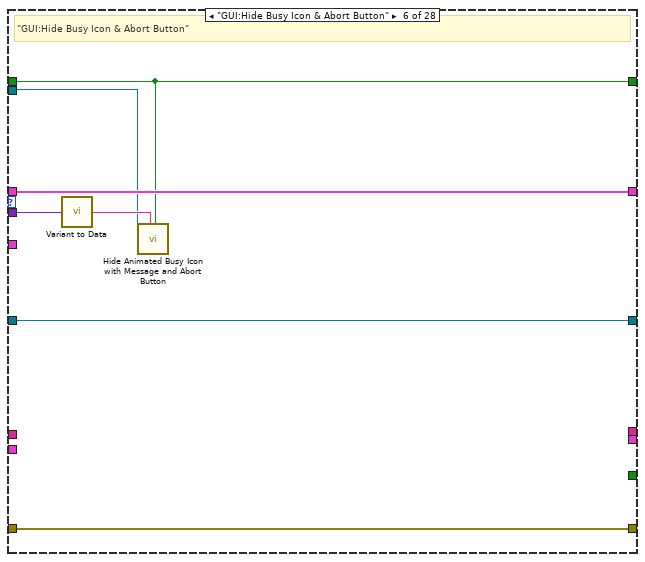
[diagram p10: hidden frame]
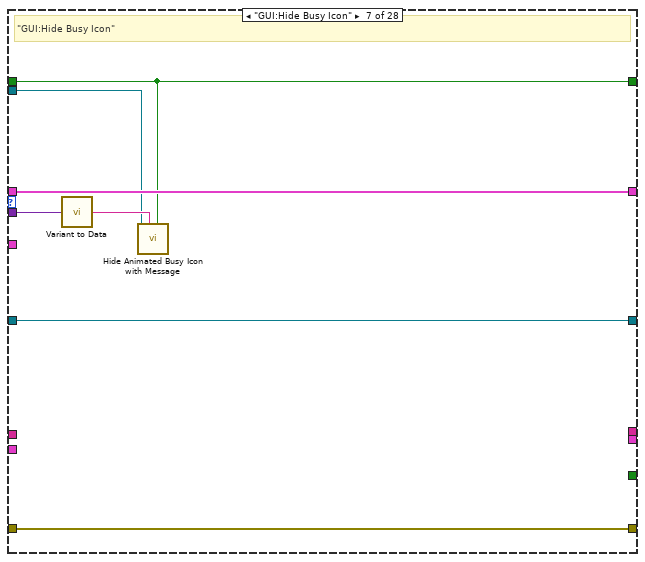
[diagram p11: hidden frame]
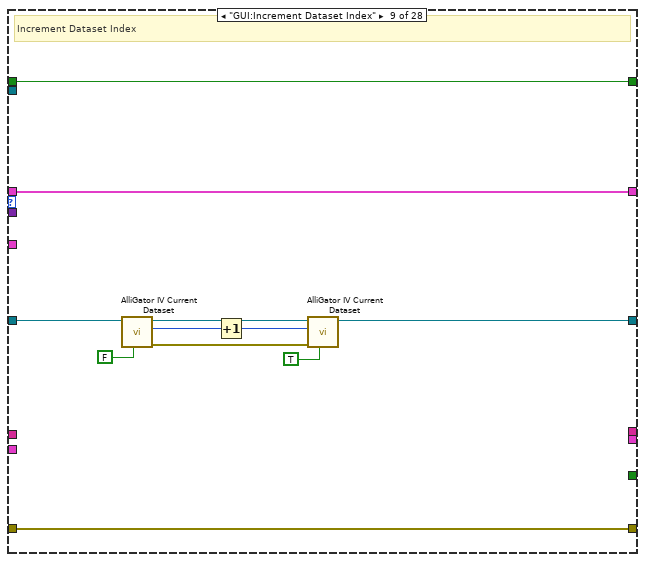
[diagram p13: hidden frame]
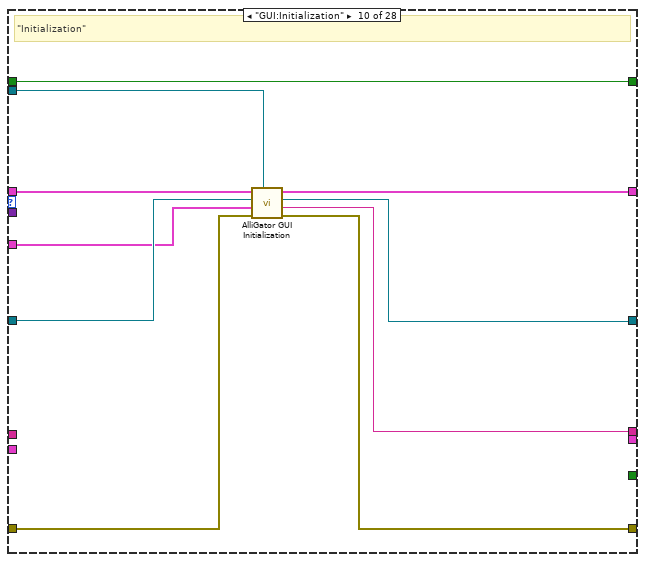
[diagram p14: hidden frame]
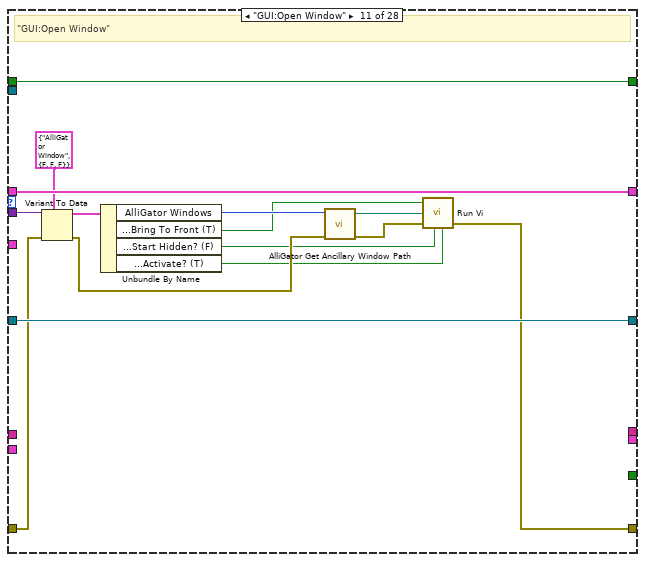
[diagram p15: hidden frame]
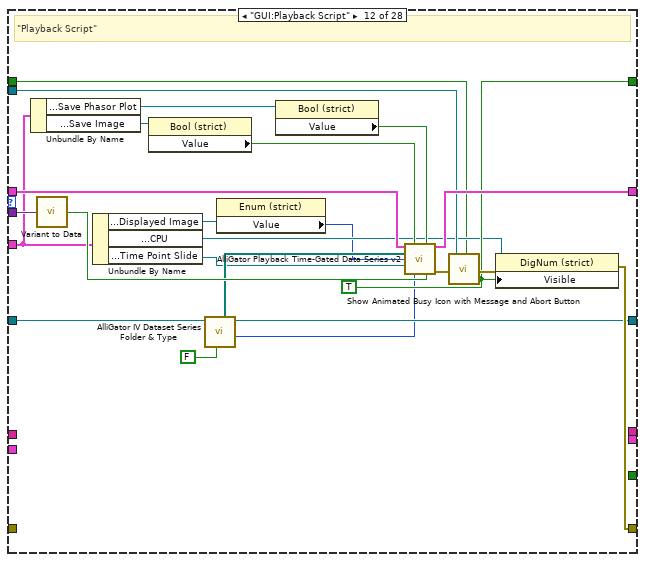
[diagram p16: hidden frame]
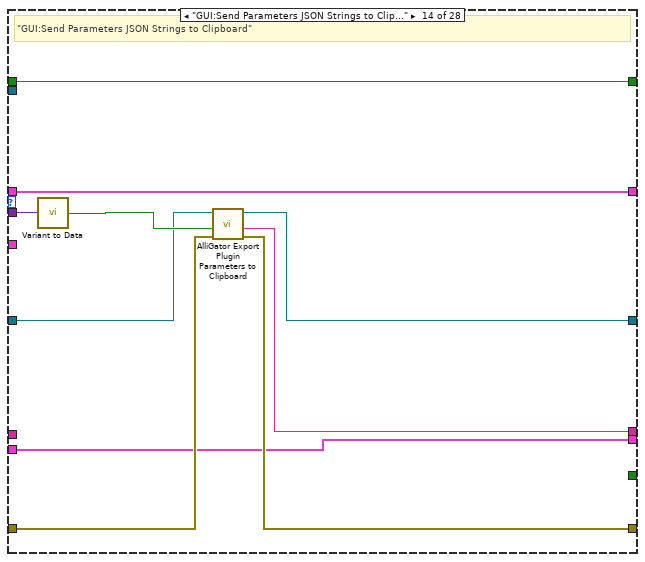
[diagram p17: hidden frame]
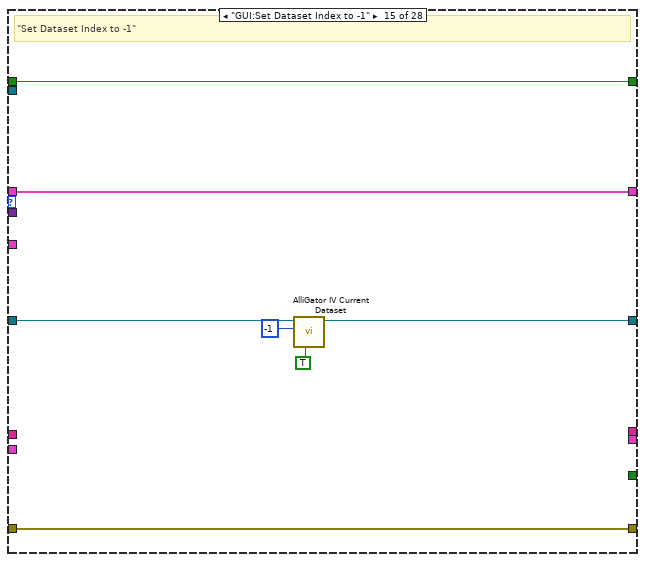
[diagram p18: hidden frame]
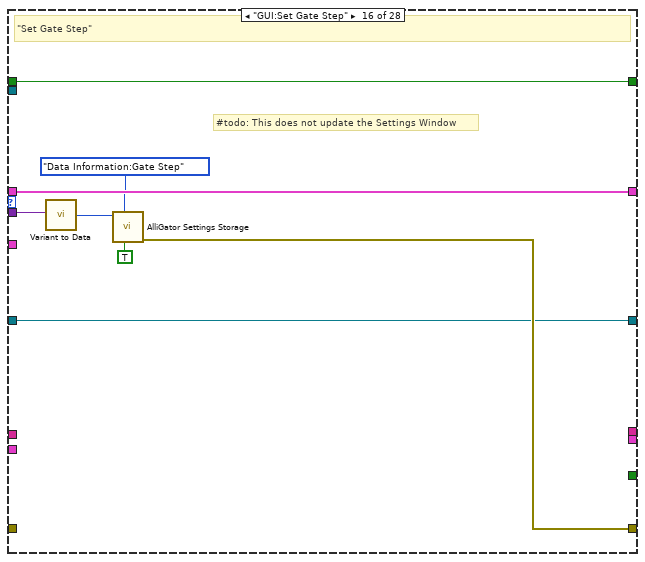
[diagram p19: hidden frame]
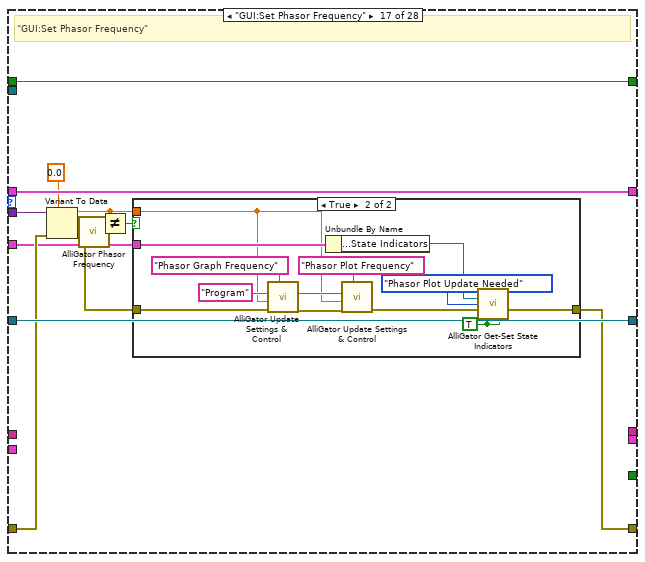
[diagram p20: hidden frame]
diagram:
  # "Author: Xavier Michalet\nCopyright 2025 REGENTS OF THE UNIVERSITY OF CALIFORNIA\n\nRedistribution and use in source and binary forms, with or without modification, are permitted provided that the following conditions are met:\n\n1. Redistributions of source code must retain the above copyright notice, this list of conditions and the following disclaimer.\n\n2. Redistributions in binary form must reproduce the above copyright notice, this list of conditions and the following disclaimer in the documentation and/or other materials provided with the distribution.\n\n3. Neither the name of the copyright holder nor the names of its contributors may be used to endorse or promote products derived from this software without specific prior written permission.\n\nTHIS SOFTWARE IS PROVIDED BY THE COPYRIGHT HOLDERS AND CONTRIBUTORS “AS IS” AND ANY EXPRESS OR IMPLIED WARRANTIES, INCLUDING, BUT NOT LIMITED TO, THE IMPLIED WARRANTIES OF MERCHANTABILITY AND FITNESS FOR A PARTICULAR PURPOSE ARE DISCLAIMED. IN NO EVENT SHALL THE COPYRIGHT HOLDER OR CONTRIBUTORS BE LIABLE FOR ANY DIRECT, INDIRECT, INCIDENTAL, SPECIAL, EXEMPLARY, OR CONSEQUENTIAL DAMAGES (INCLUDING, BUT NOT LIMITED TO, PROCUREMENT OF SUBSTITUTE GOODS OR SERVICES; LOSS OF USE, DATA, OR PROFITS; OR BUSINESS INTERRUPTION) HOWEVER CAUSED AND ON ANY THEORY OF LIABILITY, WHETHER IN CONTRACT, STRICT LIABILITY, OR TORT (INCLUDING NEGLIGENCE OR OTHERWISE) ARISING IN ANY WAY OUT OF THE USE OF THIS SOFTWARE, EVEN IF ADVISED OF THE POSSIBILITY OF SUCH DAMAGE."
  n1 = global read "AlliGator Globals.vi" "Alligator version"() -> (w7:string)
  n2 = call "Message Style.vi"() -> ("Message Formatting"=w5:T2)
  n3 = case shown="\"GUI:Quit\"" "AlliGator Q Event in" {
    tunnel: [_ _ _ _ _ _ _ _ _ _ _ _ TRUE _ _ _ _ _ _ _ _ _ _ _ _ _ _ _] -> w8
    tunnel: "Data" -> [_ _ _ _ w115 w123 w129 _ _ _ w167 w194 _ w235 _ w250 w261 w289 w294 w302 _ _ w343 w363 w369 w389 w395 w403]
    tunnel: "AlliGator Q Elements in" -> [w22 w42 w74 w103 w111 w125 w132 w136 w147 w156 w172 w196 _ w237 w244 w252 w264 w291 w298 w305 w313 w325 w342 w362 w374 w387 w399 w409]
    tunnel: [w22 w42 w74 w103 w112 w125 w132 w136 w147 w155 w172 w195 T4[] [] ("Named Q Element") w237 w244 w252 w264 w291 w298 w305 w313 w325 w341 w362 w373 w386 w399 w409] -> w10
    tunnel: "VI in" -> [_ w46 w59 _ _ w121 w127 _ _ w154 _ w189 w224 _ _ _ _ _ w292 w300 w306 _ _ _ _ _ _ _]
    tunnel: w7 -> [_ _ _ _ _ _ _ _ _ _ _ _ w223 _ _ _ _ _ _ _ _ _ _ _ _ _ _ _]
    tunnel: [w21 w45 w57 w101 w118 w120 w126 w135 w146 w157 w171 w183 w222 w236 w243 w251 w263 w290 w297 w299 w308 w324 w335 w358 w366 w390 w398 w408] -> w6
    tunnel: "Script" -> [w21 _ w56 w101 w118 w120 w126 w135 w146 w157 w171 w173 w222 w236 w243 w251 w263 w290 w297 w299 _ w324 w335 w358 w366 w390 w398 w408]
    tunnel: "error in (no error)" -> [w20 _ w55 w100 _ w119 w131 w134 w145 w153 w159 _ _ w230 w242 _ w260 _ w296 w304 w312 w323 _ w357 _ _ w397 w407]
    tunnel: [w20 w36 w72 w100 w110 w119 w131 w134 w145 w152 w158 w184 w213 w231 w242 w246 w257 w280 w296 w304 w307 w323 w334 w357 w365 w380 w397 w407] -> w15
    tunnel: "AlliGator Ctrl Refnums" -> [_ w30 w67 w99 _ _ _ _ _ w149 _ w188 w208 _ _ _ w256 w286 _ _ _ _ _ w356 _ w379 _ _]
    tunnel: "AlliGator IV DVR" -> [w19 w27 w64 w96 w109 w124 w130 w133 w144 w151 w170 w181 w207 w233 w241 w245 w262 w279 w295 w303 w311 w322 w331 w352 w364 w377 w396 w406]
    tunnel: [w19 w27 w64 w91 w107 w124 w130 w133 w142 w150 w170 w180 w207 w232 w240 w245 w262 w279 w295 w303 w310 w320 w330 w348 w364 w378 w396 w406] -> w18
    tunnel: [_ w25 w63 _ _ _ _ _ _ w148 _ _ w206 w229 _ _ _ _ _ _ _ _ _ _ _ _ _ _] -> w2
    tunnel: [_ w23 w62 _ _ _ _ _ _ _ _ _ w205 w228 _ _ _ _ _ _ _ _ _ _ _ _ _ _] -> w3
    tunnel: w5 -> [_ w23 w62 _ _ _ _ _ _ _ _ _ w205 w228 _ _ _ _ _ _ _ _ _ _ _ _ _ _]
    frame "---- GUI ----", Default {
      # "\"---- GUI ----\""
    }
    frame "GUI:Abort" {
      w45 = FALSE  # Script
      w41 = TRUE ("Get(F)/Set")
      w38 = FALSE ("Visible")
      # "\"Abort\""
      n4 = Unbundle By Name(w30) -> ("Other AlliGator Ctrl Refnums.CPU"=w29:refnum<vi>)
      n5 = call "AlliGator Settings Storage.vi"("AlliGator Settings List"=AlliGator_Settings_List."Miscellaneous:Beep after Script") -> ("Error Out"=w47:errorcluster, "Variant Data out"=w49:variant)  [unwired: 9 in]
      n6 = global write "AlliGator Abort.vi" "Abort?"(w38) -> ()
      n7 = call-poly "Variant to Data.vi"("Variant"=w49) -> ("Value"=w48:bool)  [unwired: 8 in]
      n8 = call "Hide Animated Busy Icon with Message and Abort Button.vi"("Message"="Script aborted...", "Target VI reference"=w46, "Error In"=w47) -> ("Error Out"=w31:errorcluster)  [unwired: 16 in]
      n9 = call "Alligator Variables Storage.vi"("Get(F)/Set"=w41, "AlliGator Variable"=AlliGator_Variables_List."GUI:Script in progress" ("Alligator Variable"), "Data in"=w38) -> ("Error Out"=w33:errorcluster)  [unwired: 6 in, 2 out]
      n10 = call "Alligator Variables Storage.vi"("Get(F)/Set"=w41, "AlliGator Variable"=AlliGator_Variables_List."GUI:Playback" ("Alligator Variable"), "Data in"=w38) -> ("Error Out"=w34:errorcluster)  [unwired: 6 in, 2 out]
      n11 = call "Alligator Variables Storage.vi"("Get(F)/Set"=w41, "AlliGator Variable"=AlliGator_Variables_List."GUI:Loop Playback" ("Alligator Variable"), "Data in"=w38) -> ("Error Out"=w35:errorcluster)  [unwired: 6 in, 2 out]
      n12 = call "Current Date & Time String (High Precision).vi"() -> ("Error Out"=w37:errorcluster, "time string"=w43:string, "date string"=w44:string)  [unwired: 8 in, 1 out]
      n13 = case shown="True" w48 {
        frame False {
        }
        frame True {
          n14 = call "Play Abort Sound.vi"() -> ()  [unwired: 27 in, 1 out]
        }
      }
      n15 = property class="DigNum (strict)"(reference=w29, "Visible"=FALSE) -> ()  [unwired: 1 in, 2 out]
      n16 = call "Alligator Variables Storage.vi"("Get(F)/Set"=w41, "AlliGator Variable"=AlliGator_Variables_List."Destination File Path" ("Alligator Variable"), "Error In"=w33, "Data in"=path "") -> ("Error Out"=w32:errorcluster)  [unwired: 5 in, 2 out]
      n17 = Format Into String(format string="Operation aborted by user on %s at %s", error in=w37, w44, w43) -> (resulting string=w25:string, error out=w24:errorcluster)  [unwired: 1 in]
      n18 = Merge Errors(w31, w32, w34, w35, w24) -> (w36:errorcluster)
    }
    frame "GUI:End Script" {
      w57 = FALSE  # Script
      w80 = TRUE ("Get(F)/Set")
      w65 = FALSE ("Visible")
      # "\"End Script\""
      n19 = call "AlliGator Settings Storage.vi"("AlliGator Settings List"=AlliGator_Settings_List."Miscellaneous:Beep after Script", "Error In"=w55) -> ("Error Out"=w75:errorcluster, "Variant Data out"=w77:variant)  [unwired: 8 in]
      n20 = Unbundle By Name(w67) -> ("Other AlliGator Ctrl Refnums.CPU"=w66:refnum<vi>)
      n21 = call-poly "Variant to Data.vi"("Variant"=w77) -> ("Value"=w76:bool)  [unwired: 8 in]
      n22 = call "Hide Animated Busy Icon with Message and Abort Button.vi"("Target VI reference"=w59, "Error In"=w75, "Abort Button Name (Abort)"="Abort") -> ("Error Out"=w73:errorcluster)  [unwired: 16 in]
      n23 = call "Alligator Variables Storage.vi"("Get(F)/Set"=w80, "AlliGator Variable"=AlliGator_Variables_List."GUI:Script in progress" ("Alligator Variable"), "Data in"=w65) -> ("Error Out"=w71:errorcluster)  [unwired: 6 in, 2 out]
      n24 = call "Alligator Variables Storage.vi"("Get(F)/Set"=w80, "AlliGator Variable"=AlliGator_Variables_List."GUI:Loop Playback" ("Alligator Variable"), "Data in"=w65) -> ("Error Out"=w69:errorcluster)  [unwired: 6 in, 2 out]
      n25 = call "Alligator Variables Storage.vi"("Get(F)/Set"=w80, "AlliGator Variable"=AlliGator_Variables_List."GUI:Playback" ("Alligator Variable"), "Data in"=w65) -> ("Error Out"=w70:errorcluster)  [unwired: 6 in, 2 out]
      n26 = call "Hide Animated Busy Icon with Message and Abort Button.vi"("Target VI reference"=w59, "Error In"=w73, "Abort Button Name (Abort)"="Abort Fit") -> ("Error Out"=w60:errorcluster)  [unwired: 16 in]
      n27 = case shown="True" w76 {
        frame False {
        }
        frame True {
          n28 = call "Play End of Task Sound.vi"() -> ()  [unwired: 27 in, 1 out]
        }
      }
      n29 = case shown="False" w56 {
        tunnel: [_ w84] -> w68
        tunnel: [_ w83] -> w63
        frame False {
        }
        frame True {
          n30 = call "Current Date & Time String (High Precision).vi"() -> ("Error Out"=w85:errorcluster, "time string"=w86:string, "date string"=w87:string)  [unwired: 8 in, 1 out]
          n31 = Format Into String(format string="Script stopped on %s at %s", error in=w85, w87, w86) -> (resulting string=w83:string, error out=w84:errorcluster)  [unwired: 1 in]
        }
      }
      n32 = property class="DigNum (strict)"(reference=w66, "Visible"=w65) -> ()  [unwired: 1 in, 2 out]
      n33 = global write "Abort Fit Global.vi" "Abort Fit"(w57) -> ()
      n34 = global write "AlliGator Abort.vi" "Abort?"(w57) -> ()
      n35 = Merge Errors(w60, w71, w70, w69, w68) -> (w72:errorcluster)
    }
    frame "GUI:End Timing" {
      # "\"End Timing\""
      n36 = Unbundle By Name(w99) -> ("Other AlliGator Ctrl Refnums.CPU"=w98:refnum<vi>)
      n37 = call "AlliGator IV Start Time.vi"("Get (F)/ Set (T)"=FALSE, "AlliGator IV DVR in"=w96) -> ("error out"=w92:errorcluster, "Start Time"=w95:dbl, "AlliGator IV DVR out"=w93:refnum<data-value>)  [unwired: 7 in]
      n38 = call <vilib>:"High Resolution Relative Seconds.vi"() -> ("relative seconds"=w94:dbl)
      n39 = Subtract(x=w94, y=w95) -> (x-y=w102:dbl)
      n40 = node(w102) -> (w97:dbl[unit])
      n41 = call "AlliGator IV Start Time.vi"("Get (F)/ Set (T)"=TRUE, "error in (no error)"=w92, "Start Time"=w94, "AlliGator IV DVR in"=w93) -> ("AlliGator IV DVR out"=w91:refnum<data-value>)  [unwired: 5 in, 2 out]
      n42 = property class="DigNum (strict)"(reference=w98, "Value"=w97) -> ()  [unwired: 1 in, 2 out]
    }
    frame "GUI:Gate Image Slide Changed" {
      # "\"Time Gate Slider Changed\""
      n43 = call-poly "Variant to Data.vi"("Variant"=w115) -> ("U16 Value"=w105:u16)  [unwired: 8 in]
      n44 = call "Alligator Variables Storage.vi"("Get(F)/Set"=TRUE, "AlliGator Variable"=AlliGator_Variables_List."X_Time Gate Slider" ("Alligator Variable"), "Data in"=w105) -> ("Error Out"=w108:errorcluster)  [unwired: 6 in, 2 out]
      n45 = call "AlliGator IV Gate Image Slide.vi"("Get (F)/ Set (T)"=TRUE, "error in (no error)"=w108, "Gate Image Slide"=w105, "AlliGator IV DVR in"=w109) -> ("error out"=w106:errorcluster, "AlliGator IV DVR out"=w107:refnum<data-value>)  [unwired: 5 in, 1 out]
      n46 = call-poly "AlliGator Add Action(s) to Stack.vi"("Elements Order in Action Stack (Default: 2 BEFORE 1)"=Alligator_Elements_Order_in_Action_Stack."Enqueue 2 AFTER 1", "Error In"=w106, "Alligator Atomic Action"=T4 {"AlliGator Q Event"=enum."Image:Update Image Profile Plots", "Data"=variant}, "Alligator Queue Element 1"=w111) -> ("Error Out"=w110:errorcluster, "Alligator Queue Element 1 (+ 2)"=w112:T4[])  [unwired: 6 in]
    }
    frame "GUI:Hide Busy Icon & Abort Button" {
      # "\"GUI:Hide Busy Icon & Abort Button\""
      n47 = call-poly "Variant to Data.vi"("Variant"=w123) -> ("String"=w122:string)  [unwired: 8 in]
      n48 = call "Hide Animated Busy Icon with Message and Abort Button.vi"("Already active? (F)"=w120, "Message"=w122, "Target VI reference"=w121) -> ()  [unwired: 16 in, 1 out]
    }
    frame "GUI:Hide Busy Icon" {
      # "\"GUI:Hide Busy Icon\""
      n49 = call-poly "Variant to Data.vi"("Variant"=w129) -> ("String"=w128:string)  [unwired: 8 in]
      n50 = call "Hide Animated Busy Icon with Message.vi"("Already active? (F)"=w126, "Message"=w128, "Target VI reference"=w127) -> ()  [unwired: 8 in, 1 out]
    }
    frame "GUI:Idle" {
      # "\"Idle\""
    }
    frame "GUI:Increment Dataset Index" {
      # "Increment Dataset Index"
      n51 = call "AlliGator IV Current Dataset.vi"("Get (F)/ Set (T)"=FALSE, "AlliGator IV DVR in"=w144) -> ("error out"=w139:errorcluster, "Current Dataset"=w141:i32, "AlliGator IV DVR out"=w143:refnum<data-value>)  [unwired: 7 in]
      n52 = Increment(x=w141) -> (x+1=w140:i32)
      n53 = call "AlliGator IV Current Dataset.vi"("Get (F)/ Set (T)"=TRUE, "error in (no error)"=w139, "Current Dataset"=w140, "AlliGator IV DVR in"=w143) -> ("AlliGator IV DVR out"=w142:refnum<data-value>)  [unwired: 5 in, 2 out]
    }
    frame "GUI:Initialization" {
      # "\"Initialization\""
      n54 = call "AlliGator GUI Initialization.vi"("VI in"=w154, "error in (no error)"=w153, "AlliGator Ctrl Refnums"=w149, "AlliGator IV DVR"=w151, "AlliGator Q Elements in"=w156) -> ("error out"=w152:errorcluster, "Message"=w148:string, "AlliGator IV DVR"=w150:refnum<data-value>, "AlliGator Q Elements out"=w155:T4[])  [unwired: 3 in]
    }
    frame "GUI:Open Window" {
      # "\"GUI:Open Window\""
      n55 = Variant To Data(error in=w159, type=T17 {"AlliGator Windows"=enum."AlliGator Window", "Open Window Options"={"Bring To Front (T)"=FALSE, "Start Hidden? (F)"=FALSE, "Activate? (T)"=FALSE}} ("output cluster"), Variant=w167) -> (data=w165:T17, error out=w163:errorcluster)
      n56 = Unbundle By Name(w165) -> ("AlliGator Windows"=w164:T18, "Open Window Options.Bring To Front (T)"=w162:bool, "Open Window Options.Start Hidden? (F)"=w161:bool, "Open Window Options.Activate? (T)"=w160:bool)
      n57 = call "AlliGator Get Ancillary Window Path.vi"("Error In"=w163, "AlliGator Window"=w164) -> ("Error Out"=w168:errorcluster, "VI Path"=w169:path)  [unwired: 8 in]
      n58 = call "Run Vi.vi"("Bring To Front (T)"=w162, "VI Path"=w169, "error in (no error)"=w168, "Start Hidden? (F)"=w161, "Activate? (T)"=w160) -> ("error out"=w158:errorcluster)  [unwired: 3 in, 1 out]
    }
    frame "GUI:Playback Script" {
      w183 = TRUE ("Visible")
      # "\"Playback Script\""
      n59 = Unbundle By Name(w188) -> ("Phasor Plot Ctrl Refnums.Save Phasor Plot"=w191:refnum<vi>, "Dataset Control References.Save Image"=w187:refnum<vi>)
      n60 = call-poly "Variant to Data.vi"("Variant"=w194) -> ("Value"=w193:bool)  [unwired: 8 in]
      n61 = Unbundle By Name(w188) -> ("Dataset Control References.Displayed Image"=w175:refnum<vi>, "Other AlliGator Ctrl Refnums.CPU"=w182:refnum<vi>, "Dataset Control References.Time Point Slide"=w176:refnum<vi>)
      n62 = property class="Bool (strict)"(reference=w187) -> ("Value"=w186:bool)  [unwired: 1 in, 2 out]
      n63 = call "AlliGator IV Dataset Series Folder & Type.vi"("Get (F)/ Set (T)"=FALSE, "AlliGator IV DVR in"=w181) -> ("AlliGator Data Series Type"=w179:T26, "AlliGator IV DVR out"=w180:refnum<data-value>, "[Time-Series Path]"=w178:path[])  [unwired: 5 in, 2 out]
      n64 = property class="Enum (strict)"(reference=w175) -> ("Value"=w174:T27)  [unwired: 1 in, 2 out]
      n65 = property class="Bool (strict)"(reference=w191) -> ("Value"=w190:bool)  [unwired: 1 in, 2 out]
      n66 = call "AlliGator Playback Time-Gated Data Series v2.vi"("Alligator Queue Elements in"=w196, "Save Image with Overlay"=w186, "Save Phasor Plot with Overlay"=w190, "Series Paths"=w178, "Type of Displayed Image"=w174, "Time Slider Refnum"=w176, "AlliGator Data Series Type"=w179, "Playback (F)/Loop (T)"=w193) -> ("Alligator Queue Elements out"=w195:T4[], "Error Out"=w192:errorcluster)  [unwired: 6 in]
      n67 = call "Show Animated Busy Icon with Message and Abort Button.vi"("Already active? (F)"=w173, "Target VI reference"=w189, "Error In"=w192) -> ("Error Out"=w185:errorcluster)  [unwired: 16 in]
      n68 = property class="DigNum (strict)"(reference=w182, error in=w185, "Visible"=w183) -> (error out=w184:errorcluster)  [unwired: 1 out]
    }
    frame "GUI:Quit" {
      # "\"Quit\""
      n69 = call "Formula Aliases Storage.vi"() -> ("Descriptions Array"=w200:string[], "Definitions Array"=w201:string[], "Aliases Array"=w202:string[])  [unwired: 8 in, 1 out]
      n70 = call "Open-Save Alias Definitions.vi"("Open (F)/ Save"=TRUE, "Descriptions Array in"=w200, "Definitions Array in"=w201, "Aliases Array in"=w202) -> ("Error Out"=w198:errorcluster)  [unwired: 3 in, 4 out]
      n71 = call "AlliGator Quit Source Image ROI Manager.vi"() -> ("Error Out"=w216:errorcluster)  [unwired: 11 in]
      n72 = call "AlliGator Quit Phasor Plot Image ROI Manager.vi"() -> ("Error Out"=w217:errorcluster)  [unwired: 11 in]
      n73 = call "AlliGator Save-Load Settings.vi"("Load(F)/Save (T)"=TRUE, "Error In"=w198, "AlliGator Refnum in"=w224) -> ("Error Out"=w215:errorcluster)  [unwired: 7 in, 1 out]
      n74 = call "AlliGator Hide Path Drop Boxes.vi"("Hide (F)/Show"=FALSE, "AlliGator Ctrl Refnums"=w208) -> ()  [unwired: 9 in, 1 out]
      n75 = Merge Errors(w215, w216, w217) -> (w214:errorcluster)
      n76 = call "Delete Notebook Backup on Quit.vi"("Main VI Name"="AlliGator" ("Sender")) -> ("Error Out"=w219:errorcluster)  [unwired: 10 in]
      n77 = call "AlliGator Clear Variables.vi"("Error In"=w214) -> ("Error Out"=w212:errorcluster, "Message"=w204:string)  [unwired: 9 in]
      n78 = call "Current Date & Time String (High Precision).vi"() -> ("time string"=w220:string, "date string"=w221:string)  [unwired: 8 in, 2 out]
      n79 = call "Embedded Progress Bar Q.vi"("Progress Bar Queue Name"="AlliGator Progress Bar Q") -> ("Progress Bar Queue"=w210:refnum<queue>)  [unwired: 6 in]
      n80 = Format Into String(format string="\nAlliGator %s stopped on %s at %s" ("initial string"), initial string=w204, w223, w221, w220) -> (resulting string=w206:string)  [unwired: 1 in, 1 out]
      n81 = Enqueue Element(queue=w210, element=T20 {"Action"="Quit", "Value"=0.0} ("Progress Bar Q Element")) -> ()  [unwired: 2 in, 3 out]
      n82 = Merge Errors(w212, w219) -> (w213:errorcluster)
    }
    frame "GUI:Send Parameters JSON Strings to Clipboard" {
      # "\"GUI:Send Parameters JSON Strings to Clipboard\""
      n83 = call-poly "Variant to Data.vi"("Variant"=w235) -> ("Value"=w234:bool)  [unwired: 8 in]
      n84 = call "AlliGator Export Plugin Parameters to Clipboard.vi"("Error In"=w230, "Parameter Names only"=w234, "AlliGator IV DVR"=w233) -> ("Error Out"=w231:errorcluster, "Message"=w229:string, "AlliGator IV DVR"=w232:refnum<data-value>)  [unwired: 6 in]
    }
    frame "GUI:Set Dataset Index to -1" {
      # "\"Set Dataset Index to -1\""
      n85 = call "AlliGator IV Current Dataset.vi"("Get (F)/ Set (T)"=TRUE, "Current Dataset"=-1, "AlliGator IV DVR in"=w241) -> ("AlliGator IV DVR out"=w240:refnum<data-value>)  [unwired: 6 in, 2 out]
    }
    frame "GUI:Set Gate Step" {
      # "#todo: This does not update the Settings Window"
      # "\"Set Gate Step\""
      n86 = call-poly "Variant to Data.vi"("Variant"=w250) -> ("Value"=w249:i32)  [unwired: 8 in]
      n87 = call "AlliGator Settings Storage.vi"("Get(F)/Set"=TRUE, "AlliGator Settings List"=AlliGator_Settings_List."Data Information:Gate Step", "Variant Data in"=w249) -> ("Error Out"=w246:errorcluster)  [unwired: 7 in, 1 out]
    }
    frame "GUI:Set Phasor Frequency" {
      # "\"GUI:Set Phasor Frequency\""
      n88 = Variant To Data(error in=w260, type=dbl[unit] 0.0 ("Phasor Frequency"), Variant=w261) -> (data=w255:dbl[unit], error out=w258:errorcluster)
      n89 = call "AlliGator Phasor Frequency.vi"() -> ("Phasor Frequency"=w254:dbl[unit])
      n90 = Not Equal?(x=w255, y=w254) -> (x != y?=w253:bool)
      n91 = case shown="True" w253 {
        tunnel: w258 -> [w265 w275]
        tunnel: [w265 w274] -> w257
        tunnel: w256 -> [_ w272]
        tunnel: w255 -> [_ w266]
        frame False {
        }
        frame True {
          w276 = TRUE ("ON/OFF")
          w268 = "Program" ("Sender")
          n92 = call "AlliGator Update Settings & Control.vi"("Control Label"="Phasor Graph Frequency", "Error In"=w275, "Value"=w266, "Sender"=w268) -> ("Error Out"=w270:errorcluster)  [unwired: 7 in]
          n93 = Unbundle By Name(w272) -> ("Other AlliGator Ctrl Refnums.State Indicators"=w271:refnum<vi>)
          n94 = call "AlliGator Update Settings & Control.vi"("Control Label"="Phasor Plot Frequency", "Error In"=w270, "Value"=w266, "Sender"=w268) -> ("Error Out"=w269:errorcluster)  [unwired: 7 in]
          n95 = call "AlliGator Get-Set State Indicators.vi"("State Indicators Refnum"=w271, "AlliGator State Indicators List"=AlliGator_State_Indicators_List."Phasor Plot Update Needed", "Error In"=w269, "ON/OFF"=w276, "Set (T)/Get"=w276) -> ("Error Out"=w274:errorcluster)  [unwired: 8 in, 2 out]
        }
      }
    }
    frame "GUI:Set State Indicator" {
      # "\"Set State Indicator\""
      n96 = Variant To Data(type=T22 {"State Indicators List"=enum."Phasor Calibration Defined", "ON/OFF"=FALSE, "# Defined IRFs"=0} ("Cluster"), Variant=w289) -> (data=w287:T22, error out=w282:errorcluster)  [unwired: 1 in]
      n97 = Unbundle By Name(w287) -> ("# Defined IRFs"=w281:i32, "State Indicators List"=w284:T21, "ON/OFF"=w283:bool)
      n98 = Unbundle By Name(w286) -> ("Other AlliGator Ctrl Refnums.State Indicators"=w285:refnum<vi>)
      n99 = call "AlliGator Get-Set State Indicators.vi"("# Defined IRFs"=w281, "State Indicators Refnum"=w285, "AlliGator State Indicators List"=w284, "Error In"=w282, "ON/OFF"=w283, "Set (T)/Get"=TRUE) -> ("Error Out"=w280:errorcluster)  [unwired: 7 in, 2 out]
    }
    frame "GUI:Show Busy Icon & Abort Button" {
      # "\"GUI:Show Busy Icon & Abort Button\""
      n100 = call-poly "Variant to Data.vi"("Variant"=w294) -> ("String"=w293:string)  [unwired: 8 in]
      n101 = call "Show Animated Busy Icon with Message and Abort Button.vi"("Message"=w293, "Target VI reference"=w292) -> ()  [unwired: 17 in, 1 out]
    }
    frame "GUI:Show Busy Icon" {
      # "\"GUI:Show Busy Icon\""
      n102 = call-poly "Variant to Data.vi"("Variant"=w302) -> ("String"=w301:string)  [unwired: 8 in]
      n103 = call "Show Animated Busy Icon with Message.vi"("Already active? (F)"=w299, "Message"=w301, "Target VI Refnum"=w300) -> ()  [unwired: 8 in, 1 out]
    }
    frame "GUI:Start Script" {
      w308 = TRUE ("Get(F)/Set")
      # "This is the only place this is set and results in a failure to process decays\nloaded in the Decay Graph if no script has been run before"
      # "\"GUI:Start Script\""
      n104 = call "Show Animated Busy Icon with Message and Abort Button.vi"("Target VI reference"=w306, "Error In"=w312) -> ("Error Out"=w307:errorcluster)  [unwired: 17 in]
      n105 = disable-structure shown="Enabled" {
        disable-tunnel: w311 -> [w317 w318]
        disable-tunnel: [w316 w318] -> w310
        frame Disabled {
          n106 = call "AlliGator IV Valid Decay.vi"("Get (F)/ Set (T)"=TRUE, "Valid Decay"=TRUE, "AlliGator IV DVR in"=w317) -> ("AlliGator IV DVR out"=w316:refnum<data-value>)  [unwired: 6 in, 2 out]
        }
        frame Enabled {
        }
      }
      n107 = call "Alligator Variables Storage.vi"("Get(F)/Set"=w308, "AlliGator Variable"=AlliGator_Variables_List."GUI:Script in progress" ("Alligator Variable"), "Data in"=w308) -> ()  [unwired: 6 in, 3 out]
    }
    frame "GUI:Start Timing" {
      # "\"Start Timing\""
      n108 = call <vilib>:"High Resolution Relative Seconds.vi"() -> ("relative seconds"=w321:dbl)
      n109 = call "AlliGator IV Start Time.vi"("Get (F)/ Set (T)"=TRUE, "Start Time"=w321, "AlliGator IV DVR in"=w322) -> ("AlliGator IV DVR out"=w320:refnum<data-value>)  [unwired: 6 in, 2 out]
    }
    frame "GUI:Time Series Slider Changed" {
      # "\"Time Series Slider Changed\""
      n110 = call-poly "Variant to Data.vi"("Variant"=w343) -> ("U16 Value"=w336:u16)  [unwired: 8 in]
      n111 = Decrement(x=w336) -> (x-1=w329:u16)
      n112 = call "AlliGator IV Dataset Series Folder & Type.vi"("Get (F)/ Set (T)"=FALSE, "AlliGator IV DVR in"=w331) -> ("error out"=w328:errorcluster, "[Time-Series Path]"=w333:path[])  [unwired: 5 in, 3 out]
      n113 = Index Array(array=w333, index=w329) -> (element=w338:path)
      n114 = call "AlliGator IV Current Dataset.vi"("Get (F)/ Set (T)"=TRUE, "error in (no error)"=w328, "Current Dataset"=w329, "AlliGator IV DVR in"=w331) -> ("error out"=w326:errorcluster, "AlliGator IV DVR out"=w330:refnum<data-value>)  [unwired: 5 in, 1 out]
      n115 = Bundle By Name(cluster=T4 {"AlliGator Q Event"=enum."Files:New Folder Selected", "Data"=variant} ("Alligator Atomic Action"), "Data"=w338) -> (w339:T4)
      n116 = call-poly "AlliGator Add Action(s) to Stack.vi"("Elements Order in Action Stack (Default: 2 BEFORE 1)"=Alligator_Elements_Order_in_Action_Stack."Enqueue 2 BEFORE 1", "Error In"=w326, "Alligator Atomic Action"=w339, "Alligator Queue Element 1"=w342) -> ("Error Out"=w334:errorcluster, "Alligator Queue Element 1 (+ 2)"=w341:T4[])  [unwired: 6 in]
    }
    frame "GUI:Time Series Slider Moved" {
      w347 = FALSE ("Get (F)/ Set (T)")
      # "we are only updating the folder name\nuntil the user releases the slider"
      # "\"Time Series Slider Moved\""
      n117 = Unbundle By Name(w356) -> ("Dataset Control References.Current Time Stamp"=w354:refnum<vi>, "Dataset Control References.Current Data"=w344:refnum<vi>)
      n118 = call "AlliGator IV Time Series Timestamps & Current Dataset.vi"("Get (F)/ Set"=w347, "AlliGator IV DVR in"=w352) -> ("error out"=w346:errorcluster, "[Time-Series Timestamps]"=w351:dbl[], "AlliGator IV DVR out"=w349:refnum<data-value>)  [unwired: 6 in, 1 out]
      n119 = call-poly "Variant to Data.vi"("Variant"=w363) -> ("U16 Value"=w359:u16)  [unwired: 8 in]
      n120 = Decrement(x=w359) -> (x-1=w360:u16)
      n121 = call "AlliGator IV Dataset Series Folder & Type.vi"("Get (F)/ Set (T)"=w347, "error in (no error)"=w346, "AlliGator IV DVR in"=w349) -> ("error out"=w345:errorcluster, "AlliGator IV DVR out"=w348:refnum<data-value>, "[Time-Series Path]"=w350:path[])  [unwired: 4 in, 2 out]
      n122 = Index Array(array=w351, index=w360) -> (element=w353:dbl)
      n123 = Index Array(array=w350, index=w360) -> (element=w361:path)
      n124 = Strip Path(path=w361) -> (name=w355:string)  [unwired: 1 out]
      n125 = property class="DigNum (strict)"(reference=w354, error in=w345, "Value"=w353) -> ()  [unwired: 2 out]
      n126 = property class="Str"(reference=w344, error in=w345, "Value"=w355) -> ()  [unwired: 2 out]
    }
    frame "GUI:Toggle Playback or Loop" {
      # "\"Toggle Playback or Loop\""
      n127 = call-poly "Variant to Data.vi"("Variant"=w369) -> ("Value"=w368:bool)  [unwired: 8 in]
      n128 = call "AlliGator Toggle (Loop) Playback.vi"("Playback (F)/Loop (T)"=w368) -> ("Error Out"=w370:errorcluster)  [unwired: 8 in]
      n129 = Bundle By Name(cluster=T4 {"AlliGator Q Event"=enum."GUI:Playback Script", "Data"=variant} ("Alligator Atomic Action"), "Data"=w368) -> (w371:T4)
      n130 = call "AlliGator Add Single Action to Stack.vi"("Elements Order in Action Stack (Default: 2 BEFORE 1)"=Alligator_Elements_Order_in_Action_Stack."Enqueue 2 BEFORE 1", "Error In"=w370, "Alligator Atomic Action"=w371, "Alligator Queue Element 1"=w374) -> ("Error Out"=w365:errorcluster, "Alligator Queue Element 1 (+ 2)"=w373:T4[])  [unwired: 6 in]
    }
    frame "GUI:Type of Displayed Image Changed" {
      # "\"Type of Displayed Image Changed\""
      n131 = Unbundle By Name(w379) -> ("Dataset Control References.Displayed Image"=w375:refnum<vi>, "Dataset Control References.Gate Image Slide"=w382:refnum<vi>)
      n132 = Variant To Data(type=AlliGator_Displayed_Image."Single Gate" ("NewVal"), Variant=w389) -> (data=w381:T23, error out=w383:errorcluster)  [unwired: 1 in]
      n133 = call "AlliGator Update Gate Image Slide.vi"("Displayed Image"=w375, "error in (no error)"=w383, "Type of Image"=w381, "Gate Image Slide refnum"=w382, "AlliGator IV DVR in"=w377) -> ("error out"=w376:errorcluster, "AlliGator IV DVR out"=w378:refnum<data-value>)  [unwired: 5 in]
      n134 = call-poly "AlliGator Add Action(s) to Stack.vi"("Elements Order in Action Stack (Default: 2 BEFORE 1)"=Alligator_Elements_Order_in_Action_Stack."Enqueue 2 BEFORE 1", "Error In"=w376, "Alligator Atomic Action"=T4 {"AlliGator Q Event"=enum."Image:Update Image Profile Plots", "Data"=variant}, "Alligator Queue Element 1"=w387) -> ("Error Out"=w380:errorcluster, "Alligator Queue Element 1 (+ 2)"=w386:T4[])  [unwired: 6 in]
    }
    frame "GUI:Start Test Script" {
      # "GUI:Start Test Script"
      n135 = call-poly "Variant to Data.vi"("Variant"=w395) -> ("String"=w394:string)  [unwired: 8 in]
      n136 = Bundle By Name(cluster=T25 {"Test String"="", "error"={"status"=FALSE, "code"=0, "source"=""}, "Status"=FALSE} ("output cluster"), "Test String"=w394) -> (w392:T25)
      n137 = call "AlliGator Test Internal Data.vi"("Test State"=T24."Store Test Name", "AlliGator Test Data"=w392) -> ()  [unwired: 8 in, 2 out]
    }
    frame "GUI:End Test Script" {
      # "\"GUI:End Test Script\""
      n138 = call-poly "Variant to Data.vi"("Variant"=w403) -> ("String"=w402:string)  [unwired: 8 in]
      n139 = Bundle By Name(cluster=T25 {"Test String"="", "error"={"status"=FALSE, "code"=0, "source"=""}, "Status"=FALSE} ("output cluster"), "Test String"=w402, "Status"=TRUE) -> (w404:T25)
      n140 = call "AlliGator Test Internal Data.vi"("Test State"=T24."Store Test Name", "AlliGator Test Data"=w404) -> ()  [unwired: 8 in, 2 out]
    }
  }
  "AlliGator IV DVR" <- w18
  "error out" <- w15
  "AlliGator Q Elements out" <- w10
  "Quit?" <- w8
  "Script?" <- w6
  n141 = call "AlliGator Package Notebook Messages.vi"("Message Formatting"=w3, "Message"=w2, "AlliGator Q Event in"="AlliGator Q Event in") -> ("[Notebook Message]"=→"[Notebook Message]":T1[])  [unwired: 8 in]
